vi "Main GNSS-w-Ntrip.vi"() -> ()   [LabVIEW 2019]
uses:
  C:/Users/WEGO/Documents/GitHub/Ycar/LabVIEW/Gmap/dll/GMap.NET.WindowsForms.dll
  Gmap/dll/GMap.NET.WindowsForms.dll
  Ctrl/ublox-ui_main.ctl
  Ctrl/gnss_config-2.ctl
  Ctrl/cmd_ini-add-read.ctl
  Ctrl/cmd_ini-RW.ctl
  Ctrl/cmd_common.ctl
  Ctrl/GNSS-Ntrip config.ctl
  Gmap/gmap_fgv-cmd.ctl
  Ctrl/cmd_RW.ctl
panel:
  out "GNSS time":string
  out "Ntrip conn":bool
  out "NMEA val":bool
  in  "main tap":T1(tab)
  in  "Serial Send Start/Stop":bool
  in  "GNSS Start/Stop":bool
  out "TM\nptn":u32(slide) scale=0.0..200.0
  in  "Local Time offset":u32=9
  in  "GMapControl":refnum<k24>(container)
  out "Sea Level":dbl
  out "N of Satellites":i32
  out "TM graph":T2(graph)=[{"TM array"=[{"Y(E)"=195478.83340938148, "X(N)"=532749.6315443226}, {"Y(E)"=195478.83340938148, "X(N)"=532749.6315443226}, {"Y(E)"=195478.83340938148, "X(N)"=532749.6315443226}, {"Y(E)"=195478.83340938148, "X(N)"=532749.6315443226}, {"Y(E)"=195478.83340938148, "X(N)"=532749.6315443226}, {"Y(E)"=195478.83340938148, "X(N)"=532749.6315443226}, {"Y(E)"=195478.83340938148, "X(N)"=532749.6315443226}, {"Y(E)"=195478.83340938148, "X(N)"=532749.6315443226}, {"Y(E)"=195478.83340938148, "X(N)"=532749.6315443226}, {"Y(E)"=195478.83340938148, "X(N)"=532749.6315443226}, {"Y(E)"=195478.80387262133, "X(N)"=532749.5945652778}, {"Y(E)"=195478.80387262133, "X(N)"=532749.5945652778}, {"Y(E)"=195478.80387262133, "X(N)"=532749.5945652778}, {"Y(E)"=195478.80387262133, "X(N)"=532749.5945652778}, {"Y(E)"=195478.80387262133, "X(N)"=532749.5945652778}, {"Y(E)"=195478.80387262133, "X(N)"=532749.5945652778}, {"Y(E)"=195478.80387262133, "X(N)"=532749.5945652778}, {"Y(E)"=195478.80387262133, "X(N)"=532749.5945652778}, {"Y(E)"=195478.80387262133, "X(N)"=532749.5945652778}, {"Y(E)"=195478.80387262133, "X(N)"=532749.5945652778}, {"Y(E)"=195478.80387262133, "X(N)"=532749.5945652778}, {"Y(E)"=195478.80387262133, "X(N)"=532749.5945652778}, {"Y(E)"=195478.80387262133, "X(N)"=532749.5945652778}, {"Y(E)"=195478.86283602339, "X(N)"=532749.4650507653}, {"Y(E)"=195478.86283602339, "X(N)"=532749.4650507653}, {"Y(E)"=195478.86283602339, "X(N)"=532749.4650507653}, {"Y(E)"=195478.86283602339, "X(N)"=532749.4650507653}, {"Y(E)"=195478.86283602339, "X(N)"=532749.4650507653}, {"Y(E)"=195478.86283602339, "X(N)"=532749.4650507653}, {"Y(E)"=195478.86283602339, "X(N)"=532749.4650507653}, {"Y(E)"=195478.86283602339, "X(N)"=532749.4650507653}, {"Y(E)"=195478.86283602339, "X(N)"=532749.4650507653}, {"Y(E)"=195478.86283602339, "X(N)"=532749.4650507653}, {"Y(E)"=195478.86283602339, "X(N)"=532749.4650507653}, {"Y(E)"=195478.86283602339, "X(N)"=532749.4650507653}, {"Y(E)"=195478.86283602339, "X(N)"=532749.4650507653}, {"Y(E)"=195478.8185809412, "X(N)"=532749.5020697443}, {"Y(E)"=195478.8185809412, "X(N)"=532749.5020697443}, {"Y(E)"=195478.8185809412, "X(N)"=532749.5020697443}, {"Y(E)"=195478.8185809412, "X(N)"=532749.5020697443}, {"Y(E)"=195478.8185809412, "X(N)"=532749.5020697443}, {"Y(E)"=195478.8185809412, "X(N)"=532749.5020697443}, {"Y(E)"=195478.8185809412, "X(N)"=532749.5020697443}, {"Y(E)"=195478.8185809412, "X(N)"=532749.5020697443}, {"Y(E)"=195478.8185809412, "X(N)"=532749.5020697443}, {"Y(E)"=195478.8185809412, "X(N)"=532749.5020697443}, {"Y(E)"=195478.8185809412, "X(N)"=532749.5020697443}, {"Y(E)"=195478.8185809412, "X(N)"=532749.5020697443}, {"Y(E)"=195478.8185809412, "X(N)"=532749.5020697443}, {"Y(E)"=195478.8333493192, "X(N)"=532749.5205592669}, {"Y(E)"=195478.8333493192, "X(N)"=532749.5205592669}, {"Y(E)"=195478.8333493192, "X(N)"=532749.5205592669}, {"Y(E)"=195478.8333493192, "X(N)"=532749.5205592669}, {"Y(E)"=195478.8333493192, "X(N)"=532749.5205592669}, {"Y(E)"=195478.8333493192, "X(N)"=532749.5205592669}, {"Y(E)"=195478.8333493192, "X(N)"=532749.5205592669}, {"Y(E)"=195478.8333493192, "X(N)"=532749.5205592669}, {"Y(E)"=195478.8333493192, "X(N)"=532749.5205592669}, {"Y(E)"=195478.8333493192, "X(N)"=532749.5205592669}, {"Y(E)"=195478.8333493192, "X(N)"=532749.5205592669}, {"Y(E)"=195478.8333493192, "X(N)"=532749.5205592669}, {"Y(E)"=195478.81854089958, "X(N)"=532749.4280797082}, {"Y(E)"=195478.81854089958, "X(N)"=532749.4280797082}, {"Y(E)"=195478.81854089958, "X(N)"=532749.4280797082}, {"Y(E)"=195478.81854089958, "X(N)"=532749.4280797082}, {"Y(E)"=195478.81854089958, "X(N)"=532749.4280797082}, {"Y(E)"=195478.81854089958, "X(N)"=532749.4280797082}, {"Y(E)"=195478.81854089958, "X(N)"=532749.4280797082}, {"Y(E)"=195478.81854089958, "X(N)"=532749.4280797082}, {"Y(E)"=195478.81854089958, "X(N)"=532749.4280797082}, {"Y(E)"=195478.81854089958, "X(N)"=532749.4280797082}, {"Y(E)"=195478.81854089958, "X(N)"=532749.4280797082}, {"Y(E)"=195478.81854089958, "X(N)"=532749.4280797082}, {"Y(E)"=195478.81854089958, "X(N)"=532749.4280797082}, {"Y(E)"=195478.8332592258, "X(N)"=532749.3540816847}, {"Y(E)"=195478.8332592258, "X(N)"=532749.3540816847}, {"Y(E)"=195478.8332592258, "X(N)"=532749.3540816847}, {"Y(E)"=195478.8332592258, "X(N)"=532749.3540816847}, {"Y(E)"=195478.8332592258, "X(N)"=532749.3540816847}, {"Y(E)"=195478.8332592258, "X(N)"=532749.3540816847}, {"Y(E)"=195478.8332592258, "X(N)"=532749.3540816847}, {"Y(E)"=195478.8332592258, "X(N)"=532749.3540816847}, {"Y(E)"=195478.8332592258, "X(N)"=532749.3540816847}, {"Y(E)"=195478.8332592258, "X(N)"=532749.3540816847}, {"Y(E)"=195478.8332592258, "X(N)"=532749.3540816847}, {"Y(E)"=195478.8332592258, "X(N)"=532749.3540816847}, {"Y(E)"=195478.8332592258, "X(N)"=532749.3540816847}, {"Y(E)"=195478.61200383154, "X(N)"=532749.5761715989}, {"Y(E)"=195478.61200383154, "X(N)"=532749.5761715989}, {"Y(E)"=195478.61200383154, "X(N)"=532749.5761715989}, {"Y(E)"=195478.61200383154, "X(N)"=532749.5761715989}, {"Y(E)"=195478.61200383154, "X(N)"=532749.5761715989}, {"Y(E)"=195478.61200383154, "X(N)"=532749.5761715989}, {"Y(E)"=195478.61200383154, "X(N)"=532749.5761715989}, {"Y(E)"=195478.61200383154, "X(N)"=532749.5761715989}, {"Y(E)"=195478.61200383154, "X(N)"=532749.5761715989}, {"Y(E)"=195478.61200383154, "X(N)"=532749.5761715989}, {"Y(E)"=195478.61200383154, "X(N)"=532749.5761715989}, {"Y(E)"=195478.61200383154, "X(N)"=532749.5761715989}, {"Y(E)"=195478.61200383154, "X(N)"=532749.5761715989}, {"Y(E)"=195478.61197379892, "X(N)"=532749.5206790727}, {"Y(E)"=195478.61197379892, "X(N)"=532749.5206790727}, {"Y(E)"=195478.61197379892, "X(N)"=532749.5206790727}, {"Y(E)"=195478.61197379892, "X(N)"=532749.5206790727}, {"Y(E)"=195478.61197379892, "X(N)"=532749.5206790727}, {"Y(E)"=195478.61197379892, "X(N)"=532749.5206790727}, {"Y(E)"=195478.61197379892, "X(N)"=532749.5206790727}, {"Y(E)"=195478.61197379892, "X(N)"=532749.5206790727}, {"Y(E)"=195478.61197379892, "X(N)"=532749.5206790727}, {"Y(E)"=195478.61197379892, "X(N)"=532749.5206790727}, {"Y(E)"=195478.61197379892, "X(N)"=532749.5206790727}, {"Y(E)"=195478.61197379892, "X(N)"=532749.5206790727}, {"Y(E)"=195478.61197379892, "X(N)"=532749.5206790727}, {"Y(E)"=195478.64144048005, "X(N)"=532749.4281755526}, {"Y(E)"=195478.64144048005, "X(N)"=532749.4281755526}, {"Y(E)"=195478.64144048005, "X(N)"=532749.4281755526}, {"Y(E)"=195478.64144048005, "X(N)"=532749.4281755526}, {"Y(E)"=195478.64144048005, "X(N)"=532749.4281755526}, {"Y(E)"=195478.64144048005, "X(N)"=532749.4281755526}, {"Y(E)"=195478.64144048005, "X(N)"=532749.4281755526}, {"Y(E)"=195478.64144048005, "X(N)"=532749.4281755526}, {"Y(E)"=195478.64144048005, "X(N)"=532749.4281755526}, {"Y(E)"=195478.64144048005, "X(N)"=532749.4281755526}, {"Y(E)"=195478.64144048005, "X(N)"=532749.4281755526}, {"Y(E)"=195478.64144048005, "X(N)"=532749.4281755526}, {"Y(E)"=195478.64144048005, "X(N)"=532749.4281755526}, {"Y(E)"=195478.56754852948, "X(N)"=532749.2432403986}, {"Y(E)"=195478.56754852948, "X(N)"=532749.2432403986}, {"Y(E)"=195478.56754852948, "X(N)"=532749.2432403986}, {"Y(E)"=195478.56754852948, "X(N)"=532749.2432403986}, {"Y(E)"=195478.56754852948, "X(N)"=532749.2432403986}, {"Y(E)"=195478.56754852948, "X(N)"=532749.2432403986}, {"Y(E)"=195478.56754852948, "X(N)"=532749.2432403986}, {"Y(E)"=195478.56754852948, "X(N)"=532749.2432403986}, {"Y(E)"=195478.56754852948, "X(N)"=532749.2432403986}, {"Y(E)"=195478.56754852948, "X(N)"=532749.2432403986}, {"Y(E)"=195478.56754852948, "X(N)"=532749.2432403986}, {"Y(E)"=195478.56754852948, "X(N)"=532749.2432403986}, {"Y(E)"=195478.56754852948, "X(N)"=532749.2432403986}, {"Y(E)"=195478.5822568451, "X(N)"=532749.1507448669}, {"Y(E)"=195478.5822568451, "X(N)"=532749.1507448669}, {"Y(E)"=195478.5822568451, "X(N)"=532749.1507448669}, {"Y(E)"=195478.5822568451, "X(N)"=532749.1507448669}, {"Y(E)"=195478.5822568451, "X(N)"=532749.1507448669}, {"Y(E)"=195478.5822568451, "X(N)"=532749.1507448669}, {"Y(E)"=195478.5822568451, "X(N)"=532749.1507448669}, {"Y(E)"=195478.5822568451, "X(N)"=532749.1507448669}, {"Y(E)"=195478.5822568451, "X(N)"=532749.1507448669}, {"Y(E)"=195478.5822568451, "X(N)"=532749.1507448669}, {"Y(E)"=195478.5822568451, "X(N)"=532749.1507448669}, {"Y(E)"=195478.5822568451, "X(N)"=532749.1507448669}, {"Y(E)"=195478.5822568451, "X(N)"=532749.1507448669}, {"Y(E)"=195478.3755095352, "X(N)"=532748.9103890732}, {"Y(E)"=195478.3755095352, "X(N)"=532748.9103890732}, {"Y(E)"=195478.3755095352, "X(N)"=532748.9103890732}, {"Y(E)"=195478.3755095352, "X(N)"=532748.9103890732}, {"Y(E)"=195478.3755095352, "X(N)"=532748.9103890732}, {"Y(E)"=195478.3755095352, "X(N)"=532748.9103890732}, {"Y(E)"=195478.3755095352, "X(N)"=532748.9103890732}, {"Y(E)"=195478.3755095352, "X(N)"=532748.9103890732}, {"Y(E)"=195478.3755095352, "X(N)"=532748.9103890732}, {"Y(E)"=195478.3755095352, "X(N)"=532748.9103890732}, {"Y(E)"=195478.3755095352, "X(N)"=532748.9103890732}, {"Y(E)"=195478.3755095352, "X(N)"=532748.9103890732}, {"Y(E)"=195478.3755095352, "X(N)"=532748.9103890732}, {"Y(E)"=195478.37543945547, "X(N)"=532748.78090651}, {"Y(E)"=195478.37543945547, "X(N)"=532748.78090651}, {"Y(E)"=195478.37543945547, "X(N)"=532748.78090651}, {"Y(E)"=195478.37543945547, "X(N)"=532748.78090651}, {"Y(E)"=195478.37543945547, "X(N)"=532748.78090651}, {"Y(E)"=195478.37543945547, "X(N)"=532748.78090651}, {"Y(E)"=195478.37543945547, "X(N)"=532748.78090651}, {"Y(E)"=195478.37543945547, "X(N)"=532748.78090651}, {"Y(E)"=195478.37543945547, "X(N)"=532748.78090651}, {"Y(E)"=195478.37543945547, "X(N)"=532748.78090651}, {"Y(E)"=195478.37543945547, "X(N)"=532748.78090651}, {"Y(E)"=195478.37543945547, "X(N)"=532748.78090651}, {"Y(E)"=195478.5082848043, "X(N)"=532748.8178296402}, {"Y(E)"=195478.5082848043, "X(N)"=532748.8178296402}, {"Y(E)"=195478.5082848043, "X(N)"=532748.8178296402}, {"Y(E)"=195478.5082848043, "X(N)"=532748.8178296402}, {"Y(E)"=195478.5082848043, "X(N)"=532748.8178296402}, {"Y(E)"=195478.5082848043, "X(N)"=532748.8178296402}, {"Y(E)"=195478.5082848043, "X(N)"=532748.8178296402}, {"Y(E)"=195478.5082848043, "X(N)"=532748.8178296402}, {"Y(E)"=195478.5082848043, "X(N)"=532748.8178296402}, {"Y(E)"=195478.5082848043, "X(N)"=532748.8178296402}, {"Y(E)"=195478.5082848043, "X(N)"=532748.8178296402}, {"Y(E)"=195478.5082848043, "X(N)"=532748.8178296402}, {"Y(E)"=195478.5082848043, "X(N)"=532748.8178296402}, {"Y(E)"=195478.7001636224, "X(N)"=532748.8547208244}, {"Y(E)"=195478.7001636224, "X(N)"=532748.8547208244}, {"Y(E)"=195478.7001636224, "X(N)"=532748.8547208244}, {"Y(E)"=195478.7001636224, "X(N)"=532748.8547208244}, {"Y(E)"=195478.7001636224, "X(N)"=532748.8547208244}, {"Y(E)"=195478.7001636224, "X(N)"=532748.8547208244}, {"Y(E)"=195478.7001636224, "X(N)"=532748.8547208244}, {"Y(E)"=195478.7001636224, "X(N)"=532748.8547208244}, {"Y(E)"=195478.7001636224, "X(N)"=532748.8547208244}, {"Y(E)"=195478.7001636224, "X(N)"=532748.8547208244}]}, {"TM array"=[{"Y(E)"=195478.60442441847, "X(N)"=532749.6892681528}, {"Y(E)"=195478.63475492285, "X(N)"=532749.6883149784}, {"Y(E)"=195478.6649657266, "X(N)"=532749.6854592166}, {"Y(E)"=195478.69493760145, "X(N)"=532749.680712138}, {"Y(E)"=195478.72455226214, "X(N)"=532749.6740924771}, {"Y(E)"=195478.7536928331, "X(N)"=532749.6656263586}, {"Y(E)"=195478.7822443098, "X(N)"=532749.6553471944}, {"Y(E)"=195478.81009401265, "X(N)"=532749.6432955518}, {"Y(E)"=195478.83713203156, "X(N)"=532749.6295189931}, {"Y(E)"=195478.86325165984, "X(N)"=532749.6140718879}, {"Y(E)"=195478.88834981524, "X(N)"=532749.5970151991}, {"Y(E)"=195478.91232744683, "X(N)"=532749.5784162417}, {"Y(E)"=195478.93508992583, "X(N)"=532749.5583484169}, {"Y(E)"=195478.95654741913, "X(N)"=532749.5368909236}, {"Y(E)"=195478.97661524382, "X(N)"=532749.5141284446}, {"Y(E)"=195478.99521420136, "X(N)"=532749.490150813}, {"Y(E)"=195479.01227089018, "X(N)"=532749.4650526576}, {"Y(E)"=195479.02771799528, "X(N)"=532749.4389330294}, {"Y(E)"=195479.04149455403, "X(N)"=532749.4118950105}, {"Y(E)"=195479.0535461966, "X(N)"=532749.3840453076}, {"Y(E)"=195479.06382536073, "X(N)"=532749.3554938309}, {"Y(E)"=195479.0722914792, "X(N)"=532749.32635326}, {"Y(E)"=195479.07891114015, "X(N)"=532749.2967385993}, {"Y(E)"=195479.0836582188, "X(N)"=532749.2667667244}, {"Y(E)"=195479.08651398055, "X(N)"=532749.2365559207}, {"Y(E)"=195479.08746715504, "X(N)"=532749.2062254163}, {"Y(E)"=195479.08651398055, "X(N)"=532749.1758949119}, {"Y(E)"=195479.0836582188, "X(N)"=532749.1456841081}, {"Y(E)"=195479.07891114015, "X(N)"=532749.1157122332}, {"Y(E)"=195479.0722914792, "X(N)"=532749.0860975726}, {"Y(E)"=195479.06382536073, "X(N)"=532749.0569570017}, {"Y(E)"=195479.0535461966, "X(N)"=532749.0284055249}, {"Y(E)"=195479.04149455403, "X(N)"=532749.000555822}, {"Y(E)"=195479.02771799528, "X(N)"=532748.9735178031}, {"Y(E)"=195479.01227089018, "X(N)"=532748.9473981749}, {"Y(E)"=195478.99521420136, "X(N)"=532748.9223000195}, {"Y(E)"=195478.97661524382, "X(N)"=532748.898322388}, {"Y(E)"=195478.95654741913, "X(N)"=532748.8755599089}, {"Y(E)"=195478.93508992583, "X(N)"=532748.8541024156}, {"Y(E)"=195478.91232744683, "X(N)"=532748.8340345909}, {"Y(E)"=195478.88834981524, "X(N)"=532748.8154356334}, {"Y(E)"=195478.86325165984, "X(N)"=532748.7983789446}, {"Y(E)"=195478.83713203156, "X(N)"=532748.7829318395}, {"Y(E)"=195478.81009401265, "X(N)"=532748.7691552808}, {"Y(E)"=195478.7822443098, "X(N)"=532748.7571036381}, {"Y(E)"=195478.7536928331, "X(N)"=532748.746824474}, {"Y(E)"=195478.72455226214, "X(N)"=532748.7383583555}, {"Y(E)"=195478.69493760145, "X(N)"=532748.7317386946}, {"Y(E)"=195478.6649657266, "X(N)"=532748.726991616}, {"Y(E)"=195478.63475492285, "X(N)"=532748.7241358542}, {"Y(E)"=195478.60442441847, "X(N)"=532748.7231826797}, {"Y(E)"=195478.5740939141, "X(N)"=532748.7241358542}, {"Y(E)"=195478.54388311034, "X(N)"=532748.726991616}, {"Y(E)"=195478.5139112355, "X(N)"=532748.7317386946}, {"Y(E)"=195478.4842965748, "X(N)"=532748.7383583555}, {"Y(E)"=195478.45515600385, "X(N)"=532748.746824474}, {"Y(E)"=195478.42660452714, "X(N)"=532748.7571036381}, {"Y(E)"=195478.3987548243, "X(N)"=532748.7691552808}, {"Y(E)"=195478.37171680538, "X(N)"=532748.7829318395}, {"Y(E)"=195478.3455971771, "X(N)"=532748.7983789446}, {"Y(E)"=195478.3204990217, "X(N)"=532748.8154356334}, {"Y(E)"=195478.29652139012, "X(N)"=532748.8340345909}, {"Y(E)"=195478.27375891112, "X(N)"=532748.8541024156}, {"Y(E)"=195478.25230141782, "X(N)"=532748.8755599089}, {"Y(E)"=195478.23223359312, "X(N)"=532748.898322388}, {"Y(E)"=195478.21363463558, "X(N)"=532748.9223000195}, {"Y(E)"=195478.19657794677, "X(N)"=532748.9473981749}, {"Y(E)"=195478.18113084167, "X(N)"=532748.9735178031}, {"Y(E)"=195478.16735428292, "X(N)"=532749.000555822}, {"Y(E)"=195478.15530264034, "X(N)"=532749.0284055249}, {"Y(E)"=195478.14502347622, "X(N)"=532749.0569570017}, {"Y(E)"=195478.13655735774, "X(N)"=532749.0860975726}, {"Y(E)"=195478.1299376968, "X(N)"=532749.1157122332}, {"Y(E)"=195478.12519061816, "X(N)"=532749.1456841081}, {"Y(E)"=195478.1223348564, "X(N)"=532749.1758949119}, {"Y(E)"=195478.1213816819, "X(N)"=532749.2062254163}, {"Y(E)"=195478.1223348564, "X(N)"=532749.2365559207}, {"Y(E)"=195478.12519061816, "X(N)"=532749.2667667244}, {"Y(E)"=195478.1299376968, "X(N)"=532749.2967385993}, {"Y(E)"=195478.13655735774, "X(N)"=532749.32635326}, {"Y(E)"=195478.14502347622, "X(N)"=532749.3554938309}, {"Y(E)"=195478.15530264034, "X(N)"=532749.3840453076}, {"Y(E)"=195478.16735428292, "X(N)"=532749.4118950105}, {"Y(E)"=195478.18113084167, "X(N)"=532749.4389330294}, {"Y(E)"=195478.19657794677, "X(N)"=532749.4650526576}, {"Y(E)"=195478.21363463558, "X(N)"=532749.490150813}, {"Y(E)"=195478.23223359312, "X(N)"=532749.5141284446}, {"Y(E)"=195478.25230141782, "X(N)"=532749.5368909236}, {"Y(E)"=195478.27375891112, "X(N)"=532749.5583484169}, {"Y(E)"=195478.29652139012, "X(N)"=532749.5784162417}, {"Y(E)"=195478.3204990217, "X(N)"=532749.5970151991}, {"Y(E)"=195478.3455971771, "X(N)"=532749.6140718879}, {"Y(E)"=195478.37171680538, "X(N)"=532749.6295189931}, {"Y(E)"=195478.3987548243, "X(N)"=532749.6432955518}, {"Y(E)"=195478.42660452714, "X(N)"=532749.6553471944}, {"Y(E)"=195478.45515600385, "X(N)"=532749.6656263586}, {"Y(E)"=195478.4842965748, "X(N)"=532749.6740924771}, {"Y(E)"=195478.5139112355, "X(N)"=532749.680712138}, {"Y(E)"=195478.54388311034, "X(N)"=532749.6854592166}, {"Y(E)"=195478.5740939141, "X(N)"=532749.6883149784}, {"Y(E)"=195478.60442441847, "X(N)"=532749.6892681528}]}, {"TM array"=[{"Y(E)"=195478.60442441847, "X(N)"=532750.2062254163}, {"Y(E)"=195478.667214938, "X(N)"=532750.2042521447}, {"Y(E)"=195478.72975765204, "X(N)"=532750.1983401176}, {"Y(E)"=195478.79180573305, "X(N)"=532750.188512667}, {"Y(E)"=195478.85311430565, "X(N)"=532750.1748085774}, {"Y(E)"=195478.91344141285, "X(N)"=532750.1572819325}, {"Y(E)"=195478.97254897116, "X(N)"=532750.1360019022}, {"Y(E)"=195479.03020371005, "X(N)"=532750.1110524688}, {"Y(E)"=195479.08617809258, "X(N)"=532750.0825320963}, {"Y(E)"=195479.14025121345, "X(N)"=532750.0505533417}, {"Y(E)"=195479.19220967076, "X(N)"=532750.0152424106}, {"Y(E)"=195479.24184840822, "X(N)"=532749.9767386591}, {"Y(E)"=195479.2889715244, "X(N)"=532749.9351940437}, {"Y(E)"=195479.3333930459, "X(N)"=532749.8907725222}, {"Y(E)"=195479.37493766125, "X(N)"=532749.843649406}, {"Y(E)"=195479.41344141285, "X(N)"=532749.7940106685}, {"Y(E)"=195479.44875234397, "X(N)"=532749.7420522113}, {"Y(E)"=195479.4807310985, "X(N)"=532749.6879790904}, {"Y(E)"=195479.50925147094, "X(N)"=532749.6320047078}, {"Y(E)"=195479.53420090437, "X(N)"=532749.5743499689}, {"Y(E)"=195479.55548093477, "X(N)"=532749.5152424106}, {"Y(E)"=195479.5730075796, "X(N)"=532749.4549153034}, {"Y(E)"=195479.5867116692, "X(N)"=532749.3936067309}, {"Y(E)"=195479.59653911978, "X(N)"=532749.3315586499}, {"Y(E)"=195479.6024511469, "X(N)"=532749.2690159358}, {"Y(E)"=195479.60442441847, "X(N)"=532749.2062254163}, {"Y(E)"=195479.6024511469, "X(N)"=532749.1434348967}, {"Y(E)"=195479.59653911978, "X(N)"=532749.0808921827}, {"Y(E)"=195479.5867116692, "X(N)"=532749.0188441017}, {"Y(E)"=195479.5730075796, "X(N)"=532748.9575355292}, {"Y(E)"=195479.55548093477, "X(N)"=532748.897208422}, {"Y(E)"=195479.53420090437, "X(N)"=532748.8381008636}, {"Y(E)"=195479.50925147094, "X(N)"=532748.7804461247}, {"Y(E)"=195479.4807310985, "X(N)"=532748.7244717422}, {"Y(E)"=195479.44875234397, "X(N)"=532748.6703986212}, {"Y(E)"=195479.41344141285, "X(N)"=532748.618440164}, {"Y(E)"=195479.37493766125, "X(N)"=532748.5688014266}, {"Y(E)"=195479.3333930459, "X(N)"=532748.5216783104}, {"Y(E)"=195479.2889715244, "X(N)"=532748.4772567889}, {"Y(E)"=195479.24184840822, "X(N)"=532748.4357121735}, {"Y(E)"=195479.19220967076, "X(N)"=532748.397208422}, {"Y(E)"=195479.14025121345, "X(N)"=532748.3618974908}, {"Y(E)"=195479.08617809258, "X(N)"=532748.3299187362}, {"Y(E)"=195479.03020371005, "X(N)"=532748.3013983638}, {"Y(E)"=195478.97254897116, "X(N)"=532748.2764489304}, {"Y(E)"=195478.91344141285, "X(N)"=532748.2551689}, {"Y(E)"=195478.85311430565, "X(N)"=532748.2376422551}, {"Y(E)"=195478.79180573305, "X(N)"=532748.2239381656}, {"Y(E)"=195478.72975765204, "X(N)"=532748.214110715}, {"Y(E)"=195478.667214938, "X(N)"=532748.2081986879}, {"Y(E)"=195478.60442441847, "X(N)"=532748.2062254163}, {"Y(E)"=195478.54163389895, "X(N)"=532748.2081986879}, {"Y(E)"=195478.4790911849, "X(N)"=532748.214110715}, {"Y(E)"=195478.4170431039, "X(N)"=532748.2239381656}, {"Y(E)"=195478.3557345313, "X(N)"=532748.2376422551}, {"Y(E)"=195478.2954074241, "X(N)"=532748.2551689}, {"Y(E)"=195478.2362998658, "X(N)"=532748.2764489304}, {"Y(E)"=195478.1786451269, "X(N)"=532748.3013983638}, {"Y(E)"=195478.12267074437, "X(N)"=532748.3299187362}, {"Y(E)"=195478.0685976235, "X(N)"=532748.3618974908}, {"Y(E)"=195478.0166391662, "X(N)"=532748.397208422}, {"Y(E)"=195477.96700042873, "X(N)"=532748.4357121735}, {"Y(E)"=195477.91987731255, "X(N)"=532748.4772567889}, {"Y(E)"=195477.87545579104, "X(N)"=532748.5216783104}, {"Y(E)"=195477.8339111757, "X(N)"=532748.5688014266}, {"Y(E)"=195477.7954074241, "X(N)"=532748.618440164}, {"Y(E)"=195477.76009649297, "X(N)"=532748.6703986212}, {"Y(E)"=195477.72811773844, "X(N)"=532748.7244717422}, {"Y(E)"=195477.699597366, "X(N)"=532748.7804461247}, {"Y(E)"=195477.67464793258, "X(N)"=532748.8381008636}, {"Y(E)"=195477.65336790218, "X(N)"=532748.897208422}, {"Y(E)"=195477.63584125735, "X(N)"=532748.9575355292}, {"Y(E)"=195477.62213716775, "X(N)"=532749.0188441017}, {"Y(E)"=195477.61230971717, "X(N)"=532749.0808921827}, {"Y(E)"=195477.60639769005, "X(N)"=532749.1434348967}, {"Y(E)"=195477.60442441847, "X(N)"=532749.2062254163}, {"Y(E)"=195477.60639769005, "X(N)"=532749.2690159358}, {"Y(E)"=195477.61230971717, "X(N)"=532749.3315586499}, {"Y(E)"=195477.62213716775, "X(N)"=532749.3936067309}, {"Y(E)"=195477.63584125735, "X(N)"=532749.4549153034}, {"Y(E)"=195477.65336790218, "X(N)"=532749.5152424106}, {"Y(E)"=195477.67464793258, "X(N)"=532749.5743499689}, {"Y(E)"=195477.699597366, "X(N)"=532749.6320047078}, {"Y(E)"=195477.72811773844, "X(N)"=532749.6879790904}, {"Y(E)"=195477.76009649297, "X(N)"=532749.7420522113}, {"Y(E)"=195477.7954074241, "X(N)"=532749.7940106685}, {"Y(E)"=195477.8339111757, "X(N)"=532749.843649406}, {"Y(E)"=195477.87545579104, "X(N)"=532749.8907725222}, {"Y(E)"=195477.91987731255, "X(N)"=532749.9351940437}, {"Y(E)"=195477.96700042873, "X(N)"=532749.9767386591}, {"Y(E)"=195478.0166391662, "X(N)"=532750.0152424106}, {"Y(E)"=195478.0685976235, "X(N)"=532750.0505533417}, {"Y(E)"=195478.12267074437, "X(N)"=532750.0825320963}, {"Y(E)"=195478.1786451269, "X(N)"=532750.1110524688}, {"Y(E)"=195478.2362998658, "X(N)"=532750.1360019022}, {"Y(E)"=195478.2954074241, "X(N)"=532750.1572819325}, {"Y(E)"=195478.3557345313, "X(N)"=532750.1748085774}, {"Y(E)"=195478.4170431039, "X(N)"=532750.188512667}, {"Y(E)"=195478.4790911849, "X(N)"=532750.1983401176}, {"Y(E)"=195478.54163389895, "X(N)"=532750.2042521447}, {"Y(E)"=195478.60442441847, "X(N)"=532750.2062254163}]}, {"TM array"=[{"Y(E)"=195478.60442441847, "X(N)"=532751.2062254163}, {"Y(E)"=195478.73000545753, "X(N)"=532751.2022788732}, {"Y(E)"=195478.8550908856, "X(N)"=532751.1904548189}, {"Y(E)"=195478.97918704763, "X(N)"=532751.1707999178}, {"Y(E)"=195479.10180419282, "X(N)"=532751.1433917385}, {"Y(E)"=195479.22245840722, "X(N)"=532751.1083384489}, {"Y(E)"=195479.34067352384, "X(N)"=532751.0657783881}, {"Y(E)"=195479.4559830016, "X(N)"=532751.0158795213}, {"Y(E)"=195479.56793176668, "X(N)"=532750.9588387763}, {"Y(E)"=195479.67607800843, "X(N)"=532750.8948812673}, {"Y(E)"=195479.77999492307, "X(N)"=532750.824259405}, {"Y(E)"=195479.879272398, "X(N)"=532750.7472519018}, {"Y(E)"=195479.97351863034, "X(N)"=532750.6641626711}, {"Y(E)"=195480.0623616733, "X(N)"=532750.5753196281}, {"Y(E)"=195480.14545090403, "X(N)"=532750.4810733958}, {"Y(E)"=195480.22245840722, "X(N)"=532750.3817959209}, {"Y(E)"=195480.29308026948, "X(N)"=532750.2778790062}, {"Y(E)"=195480.35703777857, "X(N)"=532750.1697327645}, {"Y(E)"=195480.4140785234, "X(N)"=532750.0577839994}, {"Y(E)"=195480.46397739026, "X(N)"=532749.9424745217}, {"Y(E)"=195480.50653745106, "X(N)"=532749.824259405}, {"Y(E)"=195480.54159074073, "X(N)"=532749.7036051906}, {"Y(E)"=195480.56899891995, "X(N)"=532749.5809880454}, {"Y(E)"=195480.5886538211, "X(N)"=532749.4568918834}, {"Y(E)"=195480.60047787533, "X(N)"=532749.3318064554}, {"Y(E)"=195480.60442441847, "X(N)"=532749.2062254163}, {"Y(E)"=195480.60047787533, "X(N)"=532749.0806443772}, {"Y(E)"=195480.5886538211, "X(N)"=532748.9555589492}, {"Y(E)"=195480.56899891995, "X(N)"=532748.8314627871}, {"Y(E)"=195480.54159074073, "X(N)"=532748.7088456419}, {"Y(E)"=195480.50653745106, "X(N)"=532748.5881914275}, {"Y(E)"=195480.46397739026, "X(N)"=532748.4699763109}, {"Y(E)"=195480.4140785234, "X(N)"=532748.3546668332}, {"Y(E)"=195480.35703777857, "X(N)"=532748.2427180681}, {"Y(E)"=195480.29308026948, "X(N)"=532748.1345718263}, {"Y(E)"=195480.22245840722, "X(N)"=532748.0306549117}, {"Y(E)"=195480.14545090403, "X(N)"=532747.9313774367}, {"Y(E)"=195480.0623616733, "X(N)"=532747.8371312044}, {"Y(E)"=195479.97351863034, "X(N)"=532747.7482881615}, {"Y(E)"=195479.879272398, "X(N)"=532747.6651989308}, {"Y(E)"=195479.77999492307, "X(N)"=532747.5881914275}, {"Y(E)"=195479.67607800843, "X(N)"=532747.5175695652}, {"Y(E)"=195479.56793176668, "X(N)"=532747.4536120562}, {"Y(E)"=195479.4559830016, "X(N)"=532747.3965713113}, {"Y(E)"=195479.34067352384, "X(N)"=532747.3466724445}, {"Y(E)"=195479.22245840722, "X(N)"=532747.3041123836}, {"Y(E)"=195479.10180419282, "X(N)"=532747.269059094}, {"Y(E)"=195478.97918704763, "X(N)"=532747.2416509148}, {"Y(E)"=195478.8550908856, "X(N)"=532747.2219960137}, {"Y(E)"=195478.73000545753, "X(N)"=532747.2101719594}, {"Y(E)"=195478.60442441847, "X(N)"=532747.2062254163}, {"Y(E)"=195478.47884337942, "X(N)"=532747.2101719594}, {"Y(E)"=195478.35375795135, "X(N)"=532747.2219960137}, {"Y(E)"=195478.22966178932, "X(N)"=532747.2416509148}, {"Y(E)"=195478.10704464413, "X(N)"=532747.269059094}, {"Y(E)"=195477.98639042972, "X(N)"=532747.3041123836}, {"Y(E)"=195477.8681753131, "X(N)"=532747.3466724445}, {"Y(E)"=195477.75286583535, "X(N)"=532747.3965713113}, {"Y(E)"=195477.64091707027, "X(N)"=532747.4536120562}, {"Y(E)"=195477.53277082852, "X(N)"=532747.5175695652}, {"Y(E)"=195477.42885391388, "X(N)"=532747.5881914275}, {"Y(E)"=195477.32957643896, "X(N)"=532747.6651989308}, {"Y(E)"=195477.2353302066, "X(N)"=532747.7482881615}, {"Y(E)"=195477.14648716364, "X(N)"=532747.8371312044}, {"Y(E)"=195477.0633979329, "X(N)"=532747.9313774367}, {"Y(E)"=195476.98639042972, "X(N)"=532748.0306549117}, {"Y(E)"=195476.91576856747, "X(N)"=532748.1345718263}, {"Y(E)"=195476.85181105838, "X(N)"=532748.2427180681}, {"Y(E)"=195476.79477031354, "X(N)"=532748.3546668332}, {"Y(E)"=195476.7448714467, "X(N)"=532748.4699763109}, {"Y(E)"=195476.7023113859, "X(N)"=532748.5881914275}, {"Y(E)"=195476.66725809622, "X(N)"=532748.7088456419}, {"Y(E)"=195476.639849917, "X(N)"=532748.8314627871}, {"Y(E)"=195476.62019501586, "X(N)"=532748.9555589492}, {"Y(E)"=195476.60837096162, "X(N)"=532749.0806443772}, {"Y(E)"=195476.60442441847, "X(N)"=532749.2062254163}, {"Y(E)"=195476.60837096162, "X(N)"=532749.3318064554}, {"Y(E)"=195476.62019501586, "X(N)"=532749.4568918834}, {"Y(E)"=195476.639849917, "X(N)"=532749.5809880454}, {"Y(E)"=195476.66725809622, "X(N)"=532749.7036051906}, {"Y(E)"=195476.7023113859, "X(N)"=532749.824259405}, {"Y(E)"=195476.7448714467, "X(N)"=532749.9424745217}, {"Y(E)"=195476.79477031354, "X(N)"=532750.0577839994}, {"Y(E)"=195476.85181105838, "X(N)"=532750.1697327645}, {"Y(E)"=195476.91576856747, "X(N)"=532750.2778790062}, {"Y(E)"=195476.98639042972, "X(N)"=532750.3817959209}, {"Y(E)"=195477.0633979329, "X(N)"=532750.4810733958}, {"Y(E)"=195477.14648716364, "X(N)"=532750.5753196281}, {"Y(E)"=195477.2353302066, "X(N)"=532750.6641626711}, {"Y(E)"=195477.32957643896, "X(N)"=532750.7472519018}, {"Y(E)"=195477.42885391388, "X(N)"=532750.824259405}, {"Y(E)"=195477.53277082852, "X(N)"=532750.8948812673}, {"Y(E)"=195477.64091707027, "X(N)"=532750.9588387763}, {"Y(E)"=195477.75286583535, "X(N)"=532751.0158795213}, {"Y(E)"=195477.8681753131, "X(N)"=532751.0657783881}, {"Y(E)"=195477.98639042972, "X(N)"=532751.1083384489}, {"Y(E)"=195478.10704464413, "X(N)"=532751.1433917385}, {"Y(E)"=195478.22966178932, "X(N)"=532751.1707999178}, {"Y(E)"=195478.35375795135, "X(N)"=532751.1904548189}, {"Y(E)"=195478.47884337942, "X(N)"=532751.2022788732}, {"Y(E)"=195478.60442441847, "X(N)"=532751.2062254163}]}, {"TM array"=[{"Y(E)"=195478.60442441847, "X(N)"=532752.2062254163}, {"Y(E)"=195478.79279597706, "X(N)"=532752.2003056016}, {"Y(E)"=195478.98042411916, "X(N)"=532752.1825695202}, {"Y(E)"=195479.16656836224, "X(N)"=532752.1530871685}, {"Y(E)"=195479.35049407996, "X(N)"=532752.1119748997}, {"Y(E)"=195479.5314754016, "X(N)"=532752.0593949652}, {"Y(E)"=195479.70879807652, "X(N)"=532751.995554874}, {"Y(E)"=195479.88176229317, "X(N)"=532751.9207065736}, {"Y(E)"=195480.04968544078, "X(N)"=532751.8351454564}, {"Y(E)"=195480.2119048034, "X(N)"=532751.7392091928}, {"Y(E)"=195480.36778017535, "X(N)"=532751.6332763993}, {"Y(E)"=195480.51669638773, "X(N)"=532751.5177651446}, {"Y(E)"=195480.65806573626, "X(N)"=532751.3931312986}, {"Y(E)"=195480.79133030074, "X(N)"=532751.259866734}, {"Y(E)"=195480.9159641468, "X(N)"=532751.1184973855}, {"Y(E)"=195481.0314754016, "X(N)"=532750.9695811732}, {"Y(E)"=195481.13740819498, "X(N)"=532750.8137058013}, {"Y(E)"=195481.2333444586, "X(N)"=532750.6514864386}, {"Y(E)"=195481.31890557587, "X(N)"=532750.483563291}, {"Y(E)"=195481.39375387615, "X(N)"=532750.3105990743}, {"Y(E)"=195481.45759396735, "X(N)"=532750.1332763993}, {"Y(E)"=195481.51017390186, "X(N)"=532749.9522950777}, {"Y(E)"=195481.55128617067, "X(N)"=532749.76836936}, {"Y(E)"=195481.58076852243, "X(N)"=532749.582225117}, {"Y(E)"=195481.59850460375, "X(N)"=532749.3945969748}, {"Y(E)"=195481.60442441847, "X(N)"=532749.2062254163}, {"Y(E)"=195481.59850460375, "X(N)"=532749.0178538577}, {"Y(E)"=195481.58076852243, "X(N)"=532748.8302257155}, {"Y(E)"=195481.55128617067, "X(N)"=532748.6440814725}, {"Y(E)"=195481.51017390186, "X(N)"=532748.4601557548}, {"Y(E)"=195481.45759396735, "X(N)"=532748.2791744332}, {"Y(E)"=195481.39375387615, "X(N)"=532748.1018517582}, {"Y(E)"=195481.31890557587, "X(N)"=532747.9288875415}, {"Y(E)"=195481.2333444586, "X(N)"=532747.760964394}, {"Y(E)"=195481.13740819498, "X(N)"=532747.5987450313}, {"Y(E)"=195481.0314754016, "X(N)"=532747.4428696594}, {"Y(E)"=195480.9159641468, "X(N)"=532747.293953447}, {"Y(E)"=195480.79133030074, "X(N)"=532747.1525840985}, {"Y(E)"=195480.65806573626, "X(N)"=532747.019319534}, {"Y(E)"=195480.51669638773, "X(N)"=532746.894685688}, {"Y(E)"=195480.36778017535, "X(N)"=532746.7791744332}, {"Y(E)"=195480.2119048034, "X(N)"=532746.6732416397}, {"Y(E)"=195480.04968544078, "X(N)"=532746.5773053762}, {"Y(E)"=195479.88176229317, "X(N)"=532746.4917442589}, {"Y(E)"=195479.70879807652, "X(N)"=532746.4168959586}, {"Y(E)"=195479.5314754016, "X(N)"=532746.3530558674}, {"Y(E)"=195479.35049407996, "X(N)"=532746.3004759329}, {"Y(E)"=195479.16656836224, "X(N)"=532746.2593636641}, {"Y(E)"=195478.98042411916, "X(N)"=532746.2298813123}, {"Y(E)"=195478.79279597706, "X(N)"=532746.212145231}, {"Y(E)"=195478.60442441847, "X(N)"=532746.2062254163}, {"Y(E)"=195478.4160528599, "X(N)"=532746.212145231}, {"Y(E)"=195478.2284247178, "X(N)"=532746.2298813123}, {"Y(E)"=195478.0422804747, "X(N)"=532746.2593636641}, {"Y(E)"=195477.858354757, "X(N)"=532746.3004759329}, {"Y(E)"=195477.67737343535, "X(N)"=532746.3530558674}, {"Y(E)"=195477.50005076043, "X(N)"=532746.4168959586}, {"Y(E)"=195477.32708654378, "X(N)"=532746.4917442589}, {"Y(E)"=195477.15916339617, "X(N)"=532746.5773053762}, {"Y(E)"=195476.99694403354, "X(N)"=532746.6732416397}, {"Y(E)"=195476.8410686616, "X(N)"=532746.7791744332}, {"Y(E)"=195476.69215244922, "X(N)"=532746.894685688}, {"Y(E)"=195476.55078310068, "X(N)"=532747.019319534}, {"Y(E)"=195476.4175185362, "X(N)"=532747.1525840985}, {"Y(E)"=195476.29288469013, "X(N)"=532747.293953447}, {"Y(E)"=195476.17737343535, "X(N)"=532747.4428696594}, {"Y(E)"=195476.07144064197, "X(N)"=532747.5987450313}, {"Y(E)"=195475.97550437835, "X(N)"=532747.760964394}, {"Y(E)"=195475.88994326108, "X(N)"=532747.9288875415}, {"Y(E)"=195475.8150949608, "X(N)"=532748.1018517582}, {"Y(E)"=195475.7512548696, "X(N)"=532748.2791744332}, {"Y(E)"=195475.6986749351, "X(N)"=532748.4601557548}, {"Y(E)"=195475.65756266628, "X(N)"=532748.6440814725}, {"Y(E)"=195475.62808031452, "X(N)"=532748.8302257155}, {"Y(E)"=195475.6103442332, "X(N)"=532749.0178538577}, {"Y(E)"=195475.60442441847, "X(N)"=532749.2062254163}, {"Y(E)"=195475.6103442332, "X(N)"=532749.3945969748}, {"Y(E)"=195475.62808031452, "X(N)"=532749.582225117}, {"Y(E)"=195475.65756266628, "X(N)"=532749.76836936}, {"Y(E)"=195475.6986749351, "X(N)"=532749.9522950777}, {"Y(E)"=195475.7512548696, "X(N)"=532750.1332763993}, {"Y(E)"=195475.8150949608, "X(N)"=532750.3105990743}, {"Y(E)"=195475.88994326108, "X(N)"=532750.483563291}, {"Y(E)"=195475.97550437835, "X(N)"=532750.6514864386}, {"Y(E)"=195476.07144064197, "X(N)"=532750.8137058013}, {"Y(E)"=195476.17737343535, "X(N)"=532750.9695811732}, {"Y(E)"=195476.29288469013, "X(N)"=532751.1184973855}, {"Y(E)"=195476.4175185362, "X(N)"=532751.259866734}, {"Y(E)"=195476.55078310068, "X(N)"=532751.3931312986}, {"Y(E)"=195476.69215244922, "X(N)"=532751.5177651446}, {"Y(E)"=195476.8410686616, "X(N)"=532751.6332763993}, {"Y(E)"=195476.99694403354, "X(N)"=532751.7392091928}, {"Y(E)"=195477.15916339617, "X(N)"=532751.8351454564}, {"Y(E)"=195477.32708654378, "X(N)"=532751.9207065736}, {"Y(E)"=195477.50005076043, "X(N)"=532751.995554874}, {"Y(E)"=195477.67737343535, "X(N)"=532752.0593949652}, {"Y(E)"=195477.858354757, "X(N)"=532752.1119748997}, {"Y(E)"=195478.0422804747, "X(N)"=532752.1530871685}, {"Y(E)"=195478.2284247178, "X(N)"=532752.1825695202}, {"Y(E)"=195478.4160528599, "X(N)"=532752.2003056016}, {"Y(E)"=195478.60442441847, "X(N)"=532752.2062254163}]}]
  in  "stop":bool
  in  "gmap center":bool
  out "GNSS data info":T3 {"HDOP" scale=0.0..10.0; "PDOP" scale=0.0..10.0; "2D Acc.m" scale=0.0..10.0; "Latitude" format="%.9f"; "Longitude" format="%.9f"; "3D Acc.m" scale=0.0..10.0}
  in  "Gmap Lon":dbl format="%.7f"
  in  "Gmap Lat":dbl format="%.7f"
  in  "gnss tm config":T4(tab)
  out "gnss mode cnt":u32[](array[numeric])
  out "Histogram Graph":cluster{i32[], dbl[]}(graph)
  in  "gnss mode check":bool
  out "Min circle R":dbl format="%.2g"
  out "Points size":i32
  out "loop count":i32
  in  "tm data reset":bool
  in  "arr limit":u32=200
  in  "Ref r size":dbl=1.0 format="%.2f"
  in  "Auto\ncenter":bool
  in  "PinDropMrkr":T5(ring)=enum."red_dot" caption="Pin Drop Marker"
  out "xcenter_TM":dbl
  out "ycenter_TM":dbl
  in  "Lat Dbclk":dbl format="%.11f"
  in  "Lon Dbclk":dbl format="%.11f"
  in  "Center \nupdate s":i32=10000
  in  "zoom":dbl(slide) scale=3.0..20.0
  out "NMEA cluster":T6
  out "Sel NMEA":string
  in  "Sel NMEA type":T7(ring)=enum."$GPGGA"
  in  "GNSS Serial cfg":T8={"Port"="COM10", "rate"=115200}
  in  "GNSS Serial delay":u32=20
  out "Raw NMEA":string
  out "Serial bufferN":u32(graph)
  in  "Data w sel":bool
  in  "baud rate":u32=9600
  in  "NMEA out port":refnum<visa-resource-name> caption="Serial Send Port"
  in  "Write delay ms":u32=900
  out "log path":string
  out "TM array":cluster{"Y(E)":dbl, "X(N)":dbl}[](array[cluster])
  out "error out":errorcluster
  in  "Ntrip accounts":u8(slide) scale=10.0..1.0
  in  "Ntrip accounts":T9(array[cluster])
  in  "update mount point":bool
  in  "Mount points":u16(ring) items=["SONP-RTCM32", "GANS-RTCM32", "GUMC-RTCM32", "DBON-RTCM32", "YONS-RTCM23", "SONP-RTCM23", "GUMC-RTCM23", "GANS-RTCM31", "YONS-CMRx", "SONP-RTCM31", "GUMC-RTCM31", "GANS-RTCM23", "DBON-RTCM23", "DBON-RTCM31", "YONS-RTCM31", "YONS-RTCM32-M5", "VRS-RTCM32-M5", "VRS-RTCM31", "VRS-CMRx", "VRS-CMRplus"]
  out "RTCM recv":string
  out "Current Ntrip client info":T10={"id"="seoul", "pwd"="seoul", "ref pt"="YONS-RTCM32-M5", "address"="gnss.eseoul.go.kr", "port "=2101}
  in  "Ntrip connect":bool
  out "SourceTable recv-str":string
  out "error out 2":errorcluster caption="error out"
  # "GNSS/GPS Test Program"
  # "ver:"
  # "Made by ybbaek https://github.com/yunbum"
  # "RLmodel GNSS-Ntrip client"
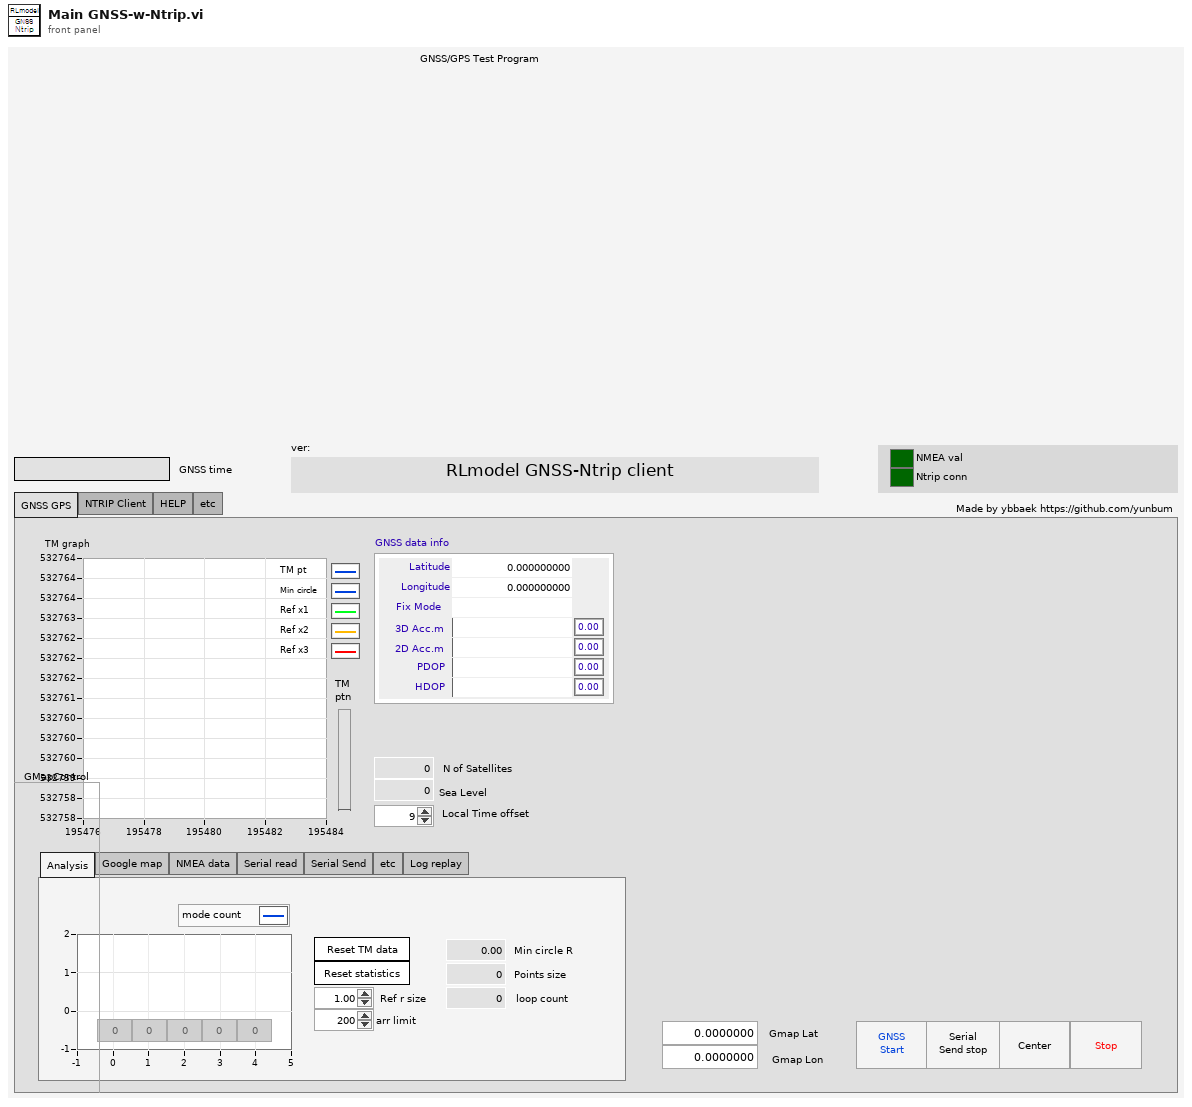
[diagram p1: front panel]
types:
  T1 = enum32{"GNSS GPS", "NTRIP Client", "HELP", "etc"}
  T2 = cluster{"TM array":cluster{"Y(E)":dbl, "X(N)":dbl}[]}[]
  T3 = typedef "ublox-ui_main.ctl" = cluster{"Latitude":dbl, "Longitude":dbl, "Fix Mode":string, "3D Acc.m":dbl, "2D Acc.m":dbl, "PDOP":dbl, "HDOP":dbl}
  T4 = enum32{"Analysis", "Google map", "NMEA data", "Serial read", "Serial Send", "etc", "Log replay"}
  T5 = enum16{"none", "arrow", "blue", "blue_small", "blue_dot", "blue_pushpin", "brown_small", "gray_small", "green", "green_small", "green_dot", "green_pushpin", "green_big_go", "yellow", "yellow_small", "yellow_dot", "yellow_big_pause", "yellow_pushpin", "lightblue", "lightblue_dot", "lightblue_pushpin", "orange", "orange_small", "orange_dot", "pink", "pink_dot", "pink_pushpin", "purple", "purple_small", "purple_dot", "purple_pushpin", "red", "red_small", "red_dot", "red_pushpin", "red_big_stop", "black_small", "white_small"}
  T6 = cluster{"GxGGA":string, "GxGSV":string, "GNRMC":string, "GxTXT":string, "GxGSA":string, "GxGLL":string}
  T7 = enum16{"$GPGSV", "$GLGSV", "$GPGGA", "$GAGSV", "$GBGSV", "$GNGLL", "$GNGGA", "$GNGSA", "$GNRMC", "$GNVTG"}
  T8 = typedef "gnss_config-2.ctl" = cluster{"Port":refnum<visa-resource-name>, "rate":u32}
  T9 = cluster{"id":string, "pwd":string, "ref pt":string, "address":string, "port ":u16}[]
  T10 = cluster{"id":string, "pwd":string, "ref pt":string, "address":string, "port ":u16}
  T11 = typedef "cmd_ini-RW.ctl" = enum16{"ini", "read", "write"}
  T12 = typedef "GNSS-Ntrip config.ctl" = cluster{"Current NtripClient Account":cluster{"id":string, "pwd":string, "ref pt":string, "address":string, "port ":u16}, "Mount points":u16, "Ref r size":dbl, "TMarr limit":i32, "Sel NMEA type":enum16{"$GPGSV", "$GLGSV", "$GPGGA", "$GAGSV", "$GBGSV", "$GNGLL", "$GNGGA", "$GNGSA", "$GNRMC", "$GNVTG"}, "Local Time offset":u32, "Write delay ms":u32, "GNSS Serial delay":u32, "Extra Serial delay":u32, "GNSS Serial cfg":T8, "Ntrip accounts":cluster{"id":string, "pwd":string, "ref pt":string, "address":string, "port ":u16}[]}
  T13 = typedef "cmd_common.ctl" = enum16{"read", "write"}
  T14 = typedef "cmd_ini-add-read.ctl" = enum16{"ini", "add", "read"}
  T15 = typedef "GNSS-Ntrip process val.ctl" = cluster{"GNSS time":string, "Ntrip conn":bool, "NMEA val":bool, "ycenter_TM":dbl, "xcenter_TM":dbl, "TM ref circles":cluster{"Y(E)":dbl, "X(N)":dbl}[], "RTCM recv-str":string, "GNSS Serail buff N":u32, "Sel NMEA type":enum16{"$GPGSV", "$GLGSV", "$GPGGA", "$GAGSV", "$GBGSV", "$GNGLL", "$GNGGA", "$GNGSA", "$GNRMC", "$GNVTG"}, "RTCM recv_sourcetable":string, "NMEA cluster":cluster{"GxGGA":string, "GxGSV":string, "GNRMC":string, "GxTXT":string, "GxGSA":string, "GxGLL":string}, "Sel NMEA str":string, "NMEA recv-str":string}
  T16 = cluster{"Gmap Lat":refnum<vi>, "Gmap Lon":refnum<vi>, "Lat Dbclk":refnum<vi>, "Lon Dbclk":refnum<vi>, "zoom":refnum<vi>, "PinDropMrkr":refnum<vi>}
  T17 = typedef "cmd_RW.ctl" = enum16{"read", "write"}
  T18 = cluster{"Ntrip tcp":bool, "GNSS serial":bool, "RTCM serial":bool, "Extra serial":bool}
  T19 = typedef "gmap_fgv-cmd.ctl" = enum16{"marker type change", "save_image", "coll of points", "zoom n center markers", "add overlay reference", "read", "zoom", "set position by keyword", "set map provider", "map provider update", "create", "add marker", "clear marker", "close"}
  T20 = typedef "NMEA.lvlib/NMEA_LatitudeDirection.ctl" = enum16{"", "North", "South"}
  T21 = typedef "NMEA.lvlib/NMEA_LongitudeDirection.ctl" = enum16{"", "East", "West"}
  T22 = typedef "NMEA.lvlib/NMEA_GPS-Quality.ctl" = enum16{"Invalid", "GPS fix (SPS)", "DGPS fix", "PPS fix", "Real Time Kinematic", "Float RTK", "estimated", "Manual input mode", "Simulation mode"}
  T23 = cluster{"$GPGGA-message_OUT":cluster{"TimeStamp":timestamp, "Latitude":dbl, "Latitude-Direction":T20, "Longitude":dbl, "Longitude-Direction":T21, "GPS-Quality":T22, "N of Satellites":i32, "HDOP":dbl, "Altitude above Mean-Sea-Level":dbl, "Geoidal separation":dbl, "Time since last DGPS update":dbl, "DGPS reference station ID":i32}}
  T24 = cluster{"NA":u32, "valid":u32, "DGPS":u32, "RTK float":u32, "RTK fixed":u32}
  T25 = cluster{"TM array":cluster{"Y(E)":dbl, "X(N)":dbl}[]}
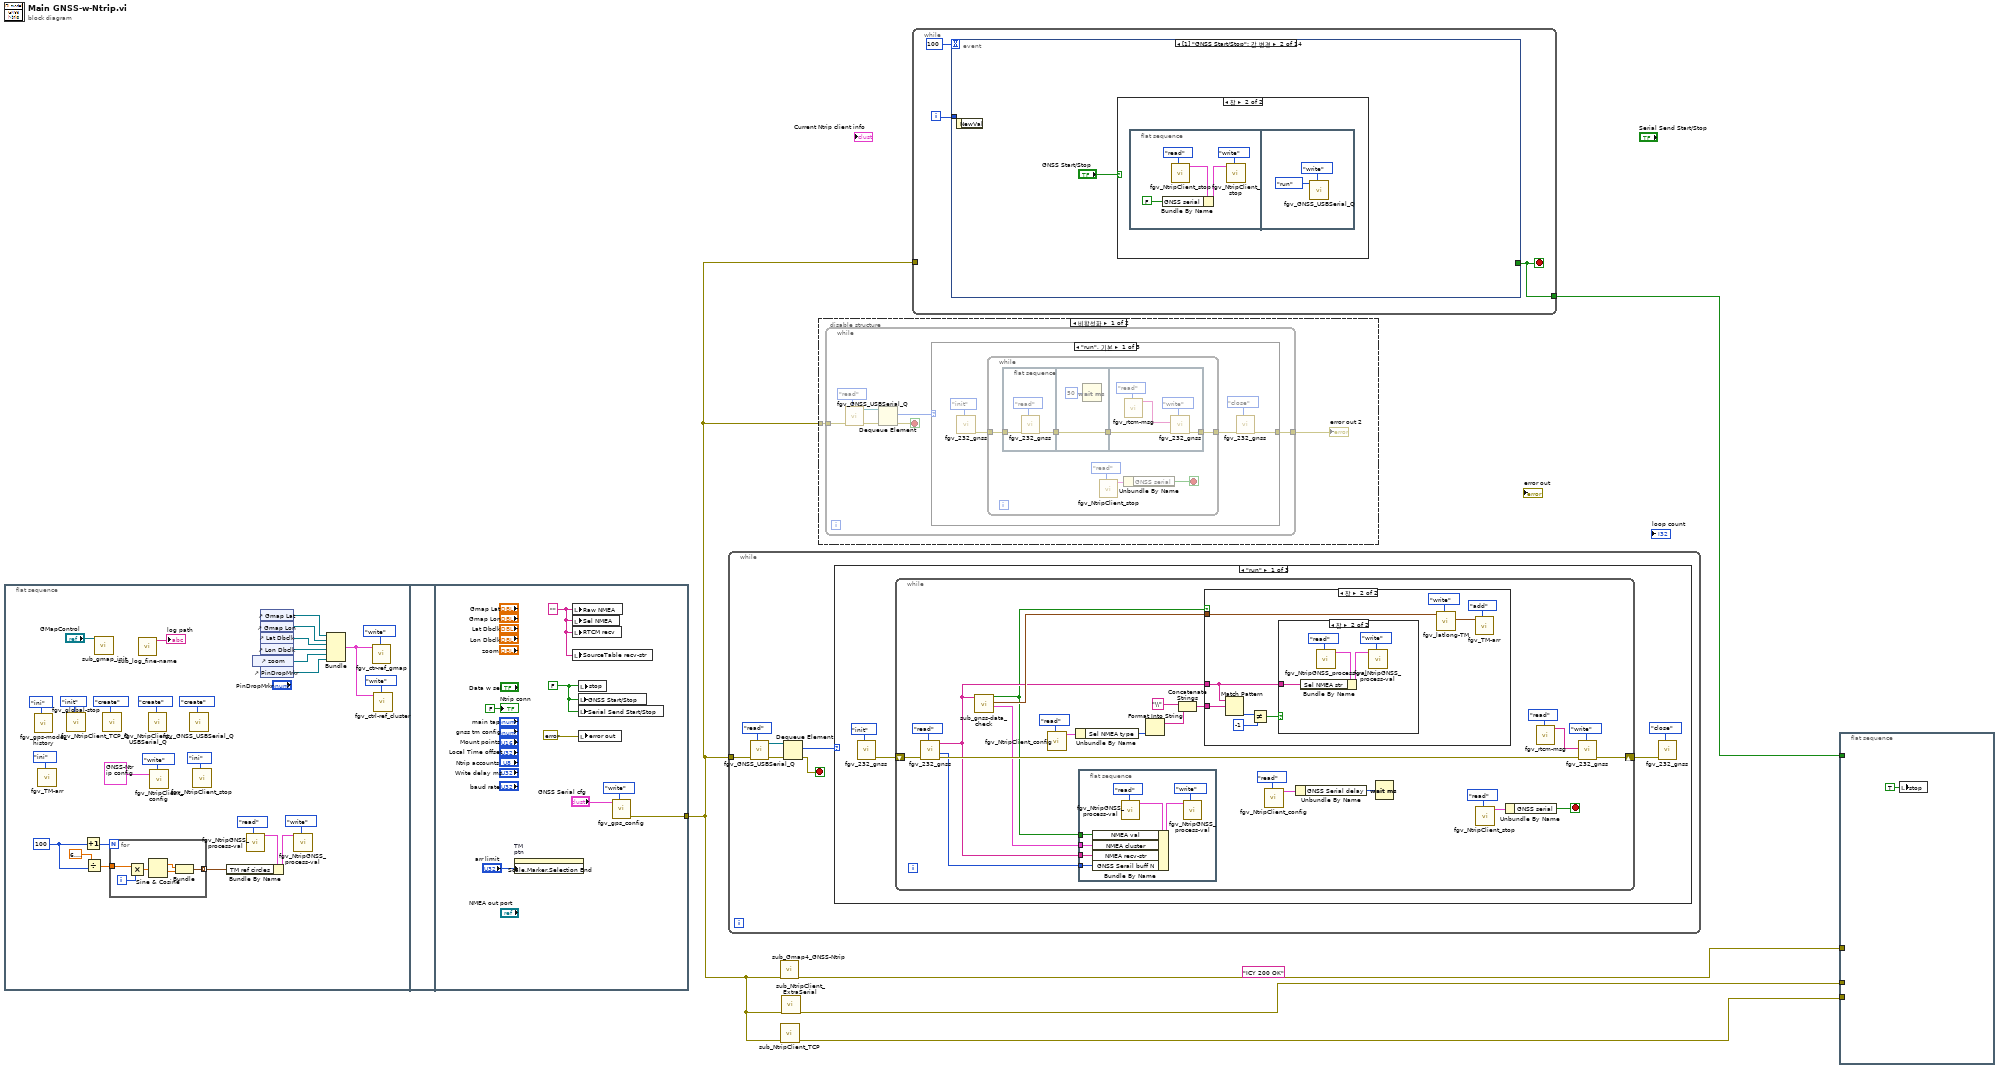
[diagram p0: block diagram]
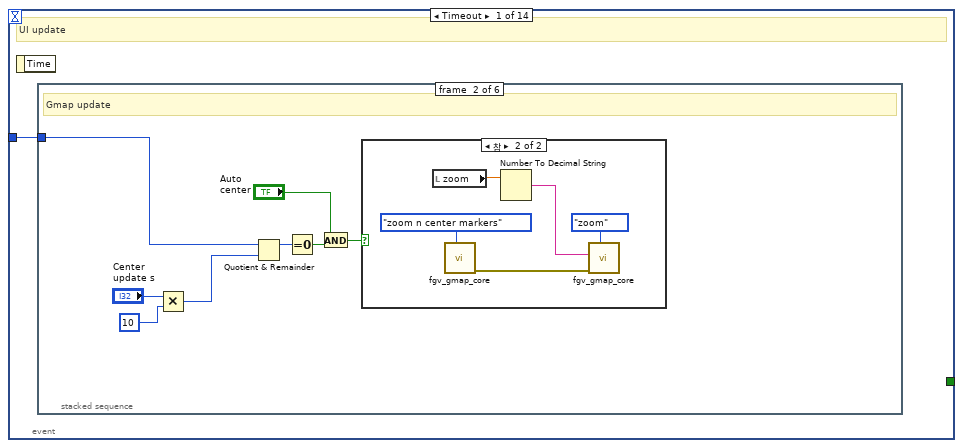
[diagram p9: hidden frame]
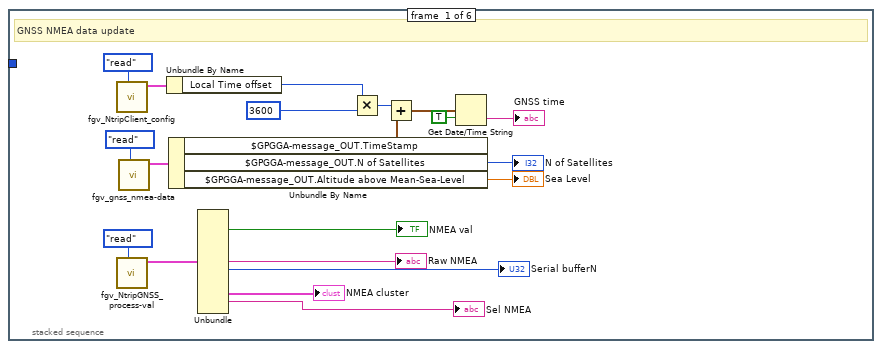
[diagram p10: hidden frame]
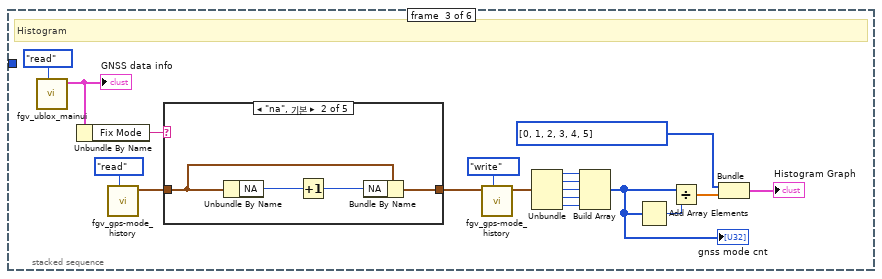
[diagram p12: hidden frame]
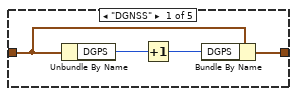
[diagram p13: hidden frame]
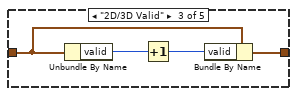
[diagram p14: hidden frame]
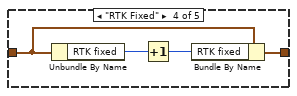
[diagram p15: hidden frame]
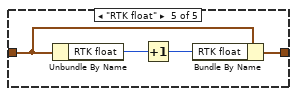
[diagram p16: hidden frame]
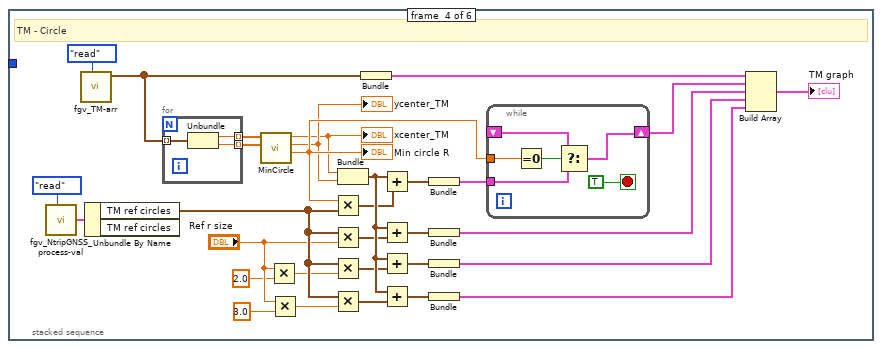
[diagram p17: hidden frame]
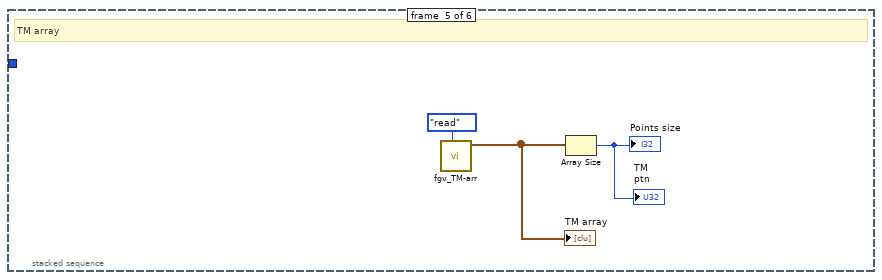
[diagram p18: hidden frame]
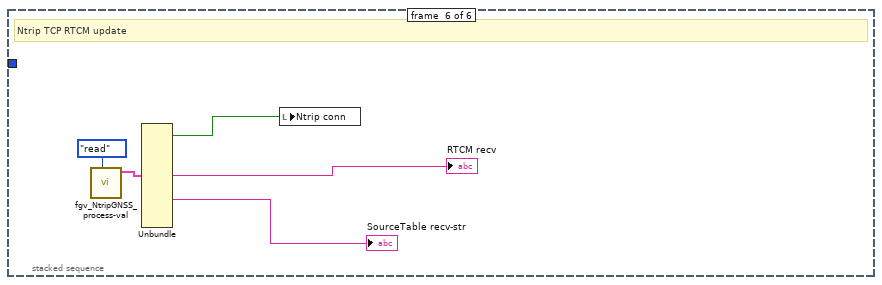
[diagram p19: hidden frame]
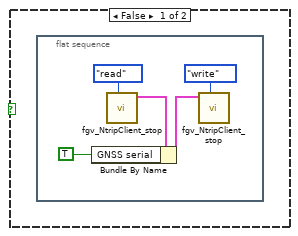
[diagram p20: hidden frame]
diagram:
  (unwired) "ICY 200 OK" ("정규식")
  n1 = flat-sequence {
    tunnel: [w47] -> w1
    frame #0 {
      w15 = 100
      n2 = call "fgv_gps-mode_history.vi"("cmd"=cmd_ini-RW."ini") -> ()  [unwired: 10 in, 1 out]
      n3 = call "fgv_TM-arr.vi"("cmd"=cmd_ini-add-read."ini") -> ()  [unwired: 10 in, 1 out]
      n4 = call "fgv_global-stop.vi"("cmd"=enum16{"init", "stop", "read"}."init") -> ()  [unwired: 10 in, 1 out]
      n5 = Increment(x=w15) -> (x+1=w17:i32)
      n6 = Divide(x=6.283185307179586, y=w15) -> (x/y=w14:dbl)
      n7 = call "sub_gmap_init.vi"("GMapControl"="GMapControl") -> ()  [unwired: 10 in, 1 out]
      n8 = call "fgv_NtripClient_TCP_Q.vi"("cmd"=enum16{"create", "write", "read", "close"}."create") -> ()  [unwired: 9 in, 2 out]
      n9 = for {
        N: w17 -> [_]
        tunnel: w14 -> [w39]
        tunnel: [w35] -> w9 mode=indexing
        i -> [w40]
        n10 = Multiply(x=w39, y=w40) -> (x*y=w38:dbl)
        n11 = Sine & Cosine(0:w38) -> (1:w37:dbl, 2:w36:dbl)
        n12 = Bundle(w37, w36) -> (w35:cluster{dbl, dbl})  [unwired: 1 in]
      }
      n13 = call "sub_log_fine-name.vi"() -> ("log path"=→"log path":string)  [unwired: 11 in]
      n14 = call "fgv_NtripClient_USBSerial_Q.vi"("cmd"=enum16{"create", "write", "read", "close"}."create") -> ()  [unwired: 9 in, 2 out]
      n15 = call "fgv_NtripClient_config.vi"("cmd"=cmd_common."write", "config val"=T12 {"Current NtripClient Account"={"id"="seoul", "pwd"="seoul", "ref pt"="YONS-RTCM32-M5", "address"="gnss.eseoul.go.kr", "port "=2101}, "Mount points"=0, "Ref r size"=1.0, "TMarr limit"=200, "Sel NMEA type"=enum."$GPGGA", "Local Time offset"=9, "Write delay ms"=900, "GNSS Serial delay"=20, "Extra Serial delay"=20, "GNSS Serial cfg"={"Port"="COM10", "rate"=115200}, "Ntrip accounts"=[]}) -> ()  [unwired: 9 in, 1 out]
      n16 = call "fgv_GNSS_USBSerial_Q.vi"("cmd"=enum16{"create", "write", "read", "close"}."create") -> ()  [unwired: 9 in, 2 out]
      n17 = call "fgv_NtripClient_stop.vi"("cmd"=cmd_ini-RW."ini") -> ()  [unwired: 10 in, 1 out]
      n18 = call "fgv_NtripGNSS_process-val.vi"("cmd"=cmd_ini-RW."read") -> ("process val out"=w13:T15)  [unwired: 10 in]
      n19 = Bundle By Name(cluster=w13, "TM ref circles"=w9) -> (w12:T15)
      n20 = control-ref of="zoom"() -> (w28:refnum<vi>)
      n21 = control-ref of="Gmap Lat"() -> (w32:refnum<vi>)
      n22 = control-ref of="Gmap Lon"() -> (w31:refnum<vi>)
      n23 = control-ref of="Lat Dbclk"() -> (w30:refnum<vi>)
      n24 = control-ref of="Lon Dbclk"() -> (w29:refnum<vi>)
      n25 = control-ref of="PinDropMrkr"() -> (w27:refnum<vi>)
      n26 = call "fgv_NtripGNSS_process-val.vi"("cmd"=cmd_ini-RW."write", "process val"=w12) -> ()  [unwired: 9 in, 1 out]
      n27 = Bundle("Gmap Lat"=w32, "Gmap Lon"=w31, "Lat Dbclk"=w30, "Lon Dbclk"=w29, "zoom"=w28, "PinDropMrkr"=w27) -> (w25:T16)  [unwired: 1 in]
      n28 = call "fgv_ctr-ref_gmap.vi"("cmd"=cmd_common."write", "ref in"=w25) -> ()  [unwired: 9 in, 1 out]
      n29 = call "fgv_ctrl-ref_cluster.vi"("cmd"=enum16{"read", "write"}."write", "ref"=w25) -> ()  [unwired: 9 in, 1 out]
    }
    frame #1 {
    }
    frame #2 {
      w42 = "" ("read raw")
      w41 = FALSE ("정지")
      n30 = property on="TM\nptn" class="Slide (엄격한)"("Scale.Marker.Selection End"="arr limit") -> ()  [unwired: 2 in, 2 out]
      n31 = local write "Raw NMEA"(w42) -> ()
      n32 = local write "Sel NMEA"(w42) -> ()
      n33 = local write "RTCM recv"(w42) -> ()
      n34 = local write "SourceTable recv-str"(w42) -> ()
      n35 = local write "GNSS Start/Stop"(w41) -> ()
      n36 = local write "Serial Send Start/Stop"(w41) -> ()
      n37 = local write "stop"(w41) -> ()
      n38 = local write "error out"(errorcluster {"status"=FALSE, "code"=0, "source"=""} ("error out")) -> ()
      n39 = call "fgv_gps_config.vi"("cmd"=enum16{"read", "write"}."write", "GNSS cfg"="GNSS Serial cfg") -> ("error out"=w47:errorcluster)  [unwired: 8 in, 1 out]
      "Ntrip conn" <- FALSE ("ntrip val")
    }
  }
  n40 = while {
    tunnel: w1 -> [w51]
    stop <- w49 stop-if-true
    n41 = call "fgv_GNSS_USBSerial_Q.vi"("cmd"=enum16{"create", "write", "read", "close"}."read", "error in"=w51) -> ("error out"=w50:errorcluster, "queue out"=w54:refnum<queue>)  [unwired: 8 in]
    n42 = Dequeue Element(queue=w54, error in (no error)=w50) -> (element=w52:enum16{"run", "check", "stop"}, error out=w49:errorcluster)  [unwired: 1 in, 2 out]
    n43 = case shown="\"run\"" w52 {
      frame "run" {
        n44 = call "fgv_232_gnss.vi"("cmd"=enum16{"init", "read", "write", "close"}."init") -> ("error out"=w57:errorcluster)  [unwired: 8 in, 2 out]
        n45 = while {
          shift-right: [w72] -> w55
          shift-left: w57 -> [w81]
          stop <- w59 stop-if-true
          n46 = call "fgv_232_gnss.vi"("cmd"=enum16{"init", "read", "write", "close"}."read", "error in"=w81) -> ("error out"=w75:errorcluster, "byte n"=w71:u32, "read_buffer"=w69:string)  [unwired: 7 in]
          n47 = call "sub_gnss-data_check.vi"("gnss str"=w69) -> ("NMEA cluster"=w68:T6, "LatLong"=w80:cluster{dbl, dbl}, "val"=w62:bool)  [unwired: 7 in, 1 out]
          n48 = call "fgv_NtripClient_config.vi"("cmd"=cmd_common."read") -> ("config val out"=w64:T12)  [unwired: 10 in]
          n49 = Unbundle By Name(w64) -> ("Sel NMEA type"=w63:T7)
          n50 = flat-sequence {
            tunnel: w71 -> [w86]
            tunnel: w69 -> [w85]
            tunnel: w68 -> [w84]
            tunnel: w62 -> [w83]
            frame #0 {
              n51 = call "fgv_NtripGNSS_process-val.vi"("cmd"=cmd_ini-RW."read") -> ("process val out"=w90:T15)  [unwired: 10 in]
              n52 = Bundle By Name(cluster=w90, "NMEA val"=w83, "NMEA cluster"=w84, "NMEA recv-str"=w85, "GNSS Serail buff N"=w86) -> (w89:T15)
              n53 = call "fgv_NtripGNSS_process-val.vi"("cmd"=cmd_ini-RW."write", "process val"=w89) -> ()  [unwired: 9 in, 1 out]
            }
          }
          n54 = Format Into String(w63) -> (resulting string=w79:string)  [unwired: 3 in, 1 out]
          n55 = Concatenate Strings("\\" ("string"), w79) -> (w77:string)
          n56 = case shown="참" w62 {
            tunnel: w69 -> [_ w93]
            tunnel: w80 -> [_ w98]
            tunnel: w77 -> [_ w97]
            frame False {
            }
            frame True {
              n57 = Match Pattern(string=w93, regular expression=w97) -> (offset past match=w96:i32)  [unwired: 1 in, 3 out]
              n58 = Not Equal?(x=w96, y=-1) -> (x != y?=w94:bool)
              n59 = case shown="참" w94 {
                tunnel: w93 -> [_ w100]
                frame False {
                }
                frame True {
                  n60 = call "fgv_NtripGNSS_process-val.vi"("cmd"=cmd_ini-RW."read") -> ("process val out"=w104:T15)  [unwired: 10 in]
                  n61 = Bundle By Name(cluster=w104, "Sel NMEA str"=w100) -> (w103:T15)
                  n62 = call "fgv_NtripGNSS_process-val.vi"("cmd"=cmd_ini-RW."write", "process val"=w103) -> ()  [unwired: 9 in, 1 out]
                }
              }
              n63 = call "fgv_latlong-TM.vi"("cmd"=enum16{"write", "read"}."write", "latlong"=w98) -> ("tm out"=w91:cluster{"YE":dbl, "XN":dbl})  [unwired: 8 in, 1 out]
              n64 = call "fgv_TM-arr.vi"("cmd"=cmd_ini-add-read."add", "TM"=w91) -> ()  [unwired: 9 in, 1 out]
            }
          }
          n65 = call "fgv_NtripClient_config.vi"("cmd"=cmd_common."read") -> ("config val out"=w66:T12)  [unwired: 10 in]
          n66 = Unbundle By Name(w66) -> ("GNSS Serial delay"=w70:u32)
          n67 = Wait (ms)(milliseconds to wait=w70) -> ()  [unwired: 1 out]
          n68 = call "fgv_NtripClient_stop.vi"("cmd"=cmd_ini-RW."read") -> ("local stops out"=w61:T18)  [unwired: 10 in]
          n69 = Unbundle By Name(w61) -> ("GNSS serial"=w59:bool)
          n70 = call "fgv_rtcm-msg.vi"("cmd"=cmd_RW."read") -> ("rtcm msg out"=w73:string)  [unwired: 10 in]
          n71 = call "fgv_232_gnss.vi"("cmd"=enum16{"init", "read", "write", "close"}."write", "error in"=w75, "write buff"=w73) -> ("error out"=w72:errorcluster)  [unwired: 6 in, 2 out]
        }
        n72 = call "fgv_232_gnss.vi"("cmd"=enum16{"init", "read", "write", "close"}."close", "error in"=w55) -> ()  [unwired: 7 in, 3 out]
      }
      frame "check" {
      }
      frame "stop", Default {
      }
    }
  }
  n73 = call "sub_Gmap4_GNSS-Ntrip.vi"("error in"=w1) -> ("error out"=w2:errorcluster)  [unwired: 10 in]
  n74 = call "sub_NtripClient_TCP.vi"("error in"=w1) -> ("error out"=w3:errorcluster)  [unwired: 10 in]
  n75 = call "sub_NtripClient_ExtraSerial.vi"("에러 입력(에러 없음)"=w1) -> ("에러 출력"=w4:errorcluster)  [unwired: 10 in]
  n76 = disable-structure shown="비활성화" {
    disable-tunnel: w1 -> [w105 _]
    frame Disabled {
      n77 = while {
        tunnel: w105 -> [w108]
        tunnel: [w107] -> w106
        stop <- w110 stop-if-true
        n78 = call "fgv_GNSS_USBSerial_Q.vi"("cmd"=enum16{"create", "write", "read", "close"}."read", "error in"=w108) -> ("error out"=w112:errorcluster, "queue out"=w111:refnum<queue>)  [unwired: 8 in]
        n79 = Dequeue Element(queue=w111, error in (no error)=w112) -> (element=w109:enum16{"run", "check", "stop"}, error out=w110:errorcluster)  [unwired: 1 in, 2 out]
        n80 = case shown="\"run\", 기본" w109 {
          tunnel: [w114 _ _] -> w107
          frame "run", Default {
            n81 = call "fgv_232_gnss.vi"("cmd"=enum16{"init", "read", "write", "close"}."init") -> ("error out"=w117:errorcluster)  [unwired: 8 in, 2 out]
            n82 = while {
              tunnel: w117 -> [w125]
              tunnel: [w122] -> w115
              stop <- w119 stop-if-true
              n83 = flat-sequence {
                tunnel: w125 -> [w127]
                tunnel: [w126] -> w123
                tunnel: [w129] -> w124
                tunnel: w123 -> [w129]
                tunnel: w124 -> [w134]
                tunnel: [w133] -> w122
                frame #0 {
                  n84 = call "fgv_232_gnss.vi"("cmd"=enum16{"init", "read", "write", "close"}."read", "error in"=w127) -> ("error out"=w126:errorcluster)  [unwired: 7 in, 2 out]
                }
                frame #1 {
                  n85 = Wait (ms)(milliseconds to wait=u32 50 ("대기 시간 (ms)")) -> ()  [unwired: 1 out]
                }
                frame #2 {
                  n86 = call "fgv_rtcm-msg.vi"("cmd"=cmd_RW."read") -> ("rtcm msg out"=w131:string)  [unwired: 10 in]
                  n87 = call "fgv_232_gnss.vi"("cmd"=enum16{"init", "read", "write", "close"}."write", "error in"=w134, "write buff"=w131) -> ("error out"=w133:errorcluster)  [unwired: 6 in, 2 out]
                }
              }
              n88 = call "fgv_NtripClient_stop.vi"("cmd"=cmd_ini-RW."read") -> ("local stops out"=w120:T18)  [unwired: 10 in]
              n89 = Unbundle By Name(w120) -> ("GNSS serial"=w119:bool)
            }
            n90 = call "fgv_232_gnss.vi"("cmd"=enum16{"init", "read", "write", "close"}."close", "error in"=w115) -> ("error out"=w114:errorcluster)  [unwired: 7 in, 2 out]
          }
          frame "check" {
          }
          frame "stop" {
          }
        }
      }
      "error out 2" <- w106
    }
    frame Enabled {
    }
  }
  n91 = while {
    tunnel: w1 -> [_]
    tunnel: [w138] -> w5
    i -> [w136]
    stop <- w138 stop-if-true
    n92 = event shown="[1] \"GNSS Start/Stop\": 값 변경" {
      selector: _ -> [_ _ _ _ _ _ _ _ _ _ _ _ _ _]
      dyn-events: _ -> [_ _ _ _ _ _ _ _ _ _ _ _ _ _]
      timeout: 100 -> [_ _ _ _ _ _ _ _ _ _ _ _ _ _]
      tunnel: [_ _ _ _ _ w281 _ _ _ _ _ _ _ _] -> w138
      tunnel: w136 -> [w139 _ _ _ _ _ _ _ _ _ _ _ _ _]
      event Timeout {
        # "UI update"
        n93 = event-data() -> ()  [unwired: 1 in, 1 out]
        n94 = stacked-sequence {
          tunnel: w139 -> [_ w160 _ _ _ _]
          frame #0 {
            # "GNSS NMEA data update"
            n95 = call "fgv_NtripClient_config.vi"("cmd"=cmd_common."read") -> ("config val out"=w152:T12)  [unwired: 10 in]
            n96 = call "fgv_NtripGNSS_process-val.vi"("cmd"=cmd_ini-RW."read") -> ("process val out"=w145:T15)  [unwired: 10 in]
            n97 = call "fgv_gnss_nmea-data.vi"("cmd"=cmd_common."read") -> ("nmea-data out"=w157:T23)  [unwired: 10 in]
            n98 = Unbundle By Name(w152) -> ("Local Time offset"=w151:u32)
            n99 = Unbundle By Name(w157) -> ("$GPGGA-message_OUT.TimeStamp"=w156:timestamp, "$GPGGA-message_OUT.N of Satellites"=→"N of Satellites":i32, "$GPGGA-message_OUT.Altitude above Mean-Sea-Level"=→"Sea Level":dbl)
            n100 = Unbundle(w145) -> ("NMEA val"=→"NMEA val":bool, "RTCM recv-str"=→"Raw NMEA":string, "GNSS Serail buff N"=→"Serial bufferN":u32, "NMEA cluster"=→"NMEA cluster":T6, "Sel NMEA str"=→"Sel NMEA":string)  [unwired: 8 out]
            n101 = Multiply(x=w151, y=u32 3600) -> (x*y=w159:u32)
            n102 = Add(x=w159, y=w156) -> (x+y=w158:timestamp)
            n103 = Get Date/Time String(seconds (now)=w158, want seconds? (F)=TRUE ("초 보이기? (거짓)")) -> (time string=→"GNSS time":string)  [unwired: 1 in, 1 out]
          }
          frame #1 {
            # "Gmap update"
            n104 = Multiply(x="Center \nupdate s", y=10) -> (x*y=w161:i32)
            n105 = Quotient & Remainder(x=w160, y=w161) -> (x-y*floor(x/y)=w165:i32)  [unwired: 1 out]
            n106 = Equal To 0?(x=w165) -> (x = 0?=w166:bool)
            n107 = And(x="Auto\ncenter", y=w166) -> (x .and. y?=w167:bool)
            n108 = case shown="참" w167 {
              frame False {
              }
              frame True {
                n109 = local read "zoom"() -> (w172:dbl)
                n110 = call "fgv_gmap_core.vi"("cmd"=gmap_fgv-cmd."zoom n center markers") -> ("error out"=w168:errorcluster)  [unwired: 7 in, 3 out]
                n111 = Number To Decimal String(number=w172) -> (decimal integer string=w171:string)  [unwired: 1 in]
                n112 = call "fgv_gmap_core.vi"(7:"cmd"=gmap_fgv-cmd."zoom" ("cmd"), "error in"=w168, 10:"cmd"=w171) -> ()  [unwired: 5 in, 4 out]
              }
            }
          }
          frame #2 {
            # "Histogram"
            n113 = call "fgv_ublox_mainui.vi"("cmd"=cmd_common."read") -> ("MainUI gnss out"=w177:T3)  [unwired: 10 in]
            "GNSS data info" <- w177
            n114 = Unbundle By Name(w177) -> ("Fix Mode"=w178:string)
            n115 = call "fgv_gps-mode_history.vi"("cmd"=cmd_ini-RW."read") -> ("data out"=w179:T24)  [unwired: 10 in]
            n116 = case shown="\"na\", 기본" w178 {
              tunnel: w179 -> [w194 w198 w202 w206 w210]
              tunnel: [w193 w197 w201 w205 w209] -> w180
              frame "DGNSS" {
                n117 = Unbundle By Name(w194) -> ("DGPS"=w192:u32)
                n118 = Increment(x=w192) -> (x+1=w191:u32)
                n119 = Bundle By Name(cluster=w194, "DGPS"=w191) -> (w193:T24)
              }
              frame "na", Default {
                n120 = Unbundle By Name(w198) -> ("NA"=w196:u32)
                n121 = Increment(x=w196) -> (x+1=w195:u32)
                n122 = Bundle By Name(cluster=w198, "NA"=w195) -> (w197:T24)
              }
              frame "2D/3D Valid" {
                n123 = Unbundle By Name(w202) -> ("valid"=w200:u32)
                n124 = Increment(x=w200) -> (x+1=w199:u32)
                n125 = Bundle By Name(cluster=w202, "valid"=w199) -> (w201:T24)
              }
              frame "RTK Fixed" {
                n126 = Unbundle By Name(w206) -> ("RTK fixed"=w204:u32)
                n127 = Increment(x=w204) -> (x+1=w203:u32)
                n128 = Bundle By Name(cluster=w206, "RTK fixed"=w203) -> (w205:T24)
              }
              frame "RTK float" {
                n129 = Unbundle By Name(w210) -> ("RTK float"=w208:u32)
                n130 = Increment(x=w208) -> (x+1=w207:u32)
                n131 = Bundle By Name(cluster=w210, "RTK float"=w207) -> (w209:T24)
              }
            }
            n132 = call "fgv_gps-mode_history.vi"("cmd"=cmd_ini-RW."write", "data"=w180) -> ("data out"=w181:T24)  [unwired: 9 in]
            n133 = Unbundle(w181) -> ("NA"=w182:u32, "valid"=w186:u32, "DGPS"=w185:u32, "RTK float"=w184:u32, "RTK fixed"=w183:u32)
            n134 = Build Array(w182, w186, w185, w184, w183) -> (w190:u32[])
            "gnss mode cnt" <- w190
            n135 = Add Array Elements(numeric array=w190) -> (sum=w188:u32)
            n136 = Divide(x=w190, y=w188) -> (x/y=w189:dbl[])
            n137 = Bundle(i32[] [0, 1, 2, 3, 4, 5], w189) -> (→"Histogram Graph":cluster{i32[], dbl[]})  [unwired: 1 in]
          }
          frame #3 {
            # "TM - Circle"
            n138 = call "fgv_NtripGNSS_process-val.vi"("cmd"=cmd_ini-RW."read") -> ("process val out"=w239:T15)  [unwired: 10 in]
            n139 = call "fgv_TM-arr.vi"("cmd"=cmd_ini-add-read."read") -> ("TM array"=w241:cluster{"Y(E)":dbl, "X(N)":dbl}[])  [unwired: 10 in]
            n140 = Unbundle By Name(w239) -> ("TM ref circles"=w240:cluster{"Y(E)":dbl, "X(N)":dbl}[])  [unwired: 1 out]
            n141 = for {
              tunnel: [w250] -> w216 mode=indexing
              tunnel: [w249] -> w217 mode=indexing
              tunnel: w241 -> [w248] mode=indexing
              n142 = Unbundle(w248) -> ("Y(E)"=w250:dbl, "X(N)"=w249:dbl)
            }
            n143 = call "MinCircle.vi"("y"=w217, "x"=w216) -> ("r"=w226:dbl, "yc"=w219:dbl, "xc"=w218:dbl)  [unwired: 6 in, 1 out]
            "xcenter_TM" <- w218
            "ycenter_TM" <- w219
            "Min circle R" <- w226
            n144 = Multiply(x="Ref r size", y=2.0) -> (x*y=w231:dbl)
            n145 = Multiply(x="Ref r size", y=3.0) -> (x*y=w212:dbl)
            n146 = Multiply(x=w226, y=w240) -> (x*y=w220:cluster{"Y(E)":dbl, "X(N)":dbl}[])
            n147 = Multiply(x=w240, y="Ref r size") -> (x*y=w230:cluster{"Y(E)":dbl, "X(N)":dbl}[])
            n148 = Multiply(x=w240, y=w231) -> (x*y=w229:cluster{"Y(E)":dbl, "X(N)":dbl}[])
            n149 = Multiply(x=w240, y=w212) -> (x*y=w232:cluster{"Y(E)":dbl, "X(N)":dbl}[])
            n150 = Bundle("xc"=w218, "yc"=w219) -> (w233:cluster{"xc":dbl, "yc":dbl})  [unwired: 1 in]
            n151 = Bundle("TM array"=w241) -> (w222:T25)  [unwired: 1 in]
            n152 = Add(x=w233, y=w220) -> (x+y=w221:cluster{dbl, dbl}[])
            n153 = Add(x=w233, y=w230) -> (x+y=w227:cluster{dbl, dbl}[])
            n154 = Add(x=w233, y=w229) -> (x+y=w235:cluster{dbl, dbl}[])
            n155 = Add(x=w233, y=w232) -> (x+y=w234:cluster{dbl, dbl}[])
            n156 = Bundle(w221) -> (w224:cluster{cluster{dbl, dbl}[]})  [unwired: 1 in]
            n157 = Bundle(w227) -> (w228:cluster{cluster{dbl, dbl}[]})  [unwired: 1 in]
            n158 = Bundle(w235) -> (w236:cluster{cluster{dbl, dbl}[]})  [unwired: 1 in]
            n159 = Bundle(w234) -> (w237:cluster{cluster{dbl, dbl}[]})  [unwired: 1 in]
            n160 = while {
              shift-right: [w242] -> w225
              shift-left: _ -> [w244]
              tunnel: w226 -> [w246]
              tunnel: w224 -> [w243]
              stop <- TRUE stop-if-true
              n161 = Equal To 0?(x=w246) -> (x = 0?=w245:bool)
              n162 = Select(t=w244, s=w245, f=w243) -> (s? t:f=w242:cluster{cluster{dbl, dbl}[]})
            }
            n163 = Build Array(w222, w225, w228, w236, w237) -> (→"TM graph":T2)
          }
          frame #4 {
            # "TM array"
            n164 = call "fgv_TM-arr.vi"("cmd"=cmd_ini-add-read."read") -> ("TM array"=w251:cluster{"Y(E)":dbl, "X(N)":dbl}[])  [unwired: 10 in]
            "TM array" <- w251
            n165 = Array Size(array=w251) -> (size(s)=→"Points size" →"TM\nptn":i32)
          }
          frame #5 {
            # "Ntrip TCP RTCM update"
            n166 = call "fgv_NtripGNSS_process-val.vi"("cmd"=cmd_ini-RW."read") -> ("process val out"=w257:T15)  [unwired: 10 in]
            n167 = Unbundle(w257) -> ("Ntrip conn"=w254:bool, "RTCM recv-str"=→"RTCM recv":string, "RTCM recv_sourcetable"=→"SourceTable recv-str":string)  [unwired: 10 out]
            n168 = local write "Ntrip conn"(w254) -> ()
          }
        }
      }
      event "GNSS Start/Stop": Value Change {
        n169 = event-data() -> ()  [unwired: 1 in, 1 out]
        n170 = case shown="참" "GNSS Start/Stop" {
          frame False {
            n171 = flat-sequence {
              frame #0 {
                n172 = call "fgv_NtripClient_stop.vi"("cmd"=cmd_ini-RW."read") -> ("local stops out"=w262:T18)  [unwired: 10 in]
                n173 = Bundle By Name(cluster=w262, "GNSS serial"=TRUE ("Ntrip tcp")) -> (w261:T18)
                n174 = call "fgv_NtripClient_stop.vi"("cmd"=cmd_ini-RW."write", "local stops"=w261) -> ()  [unwired: 9 in, 1 out]
              }
            }
          }
          frame True {
            n175 = flat-sequence {
              frame #0 {
                n176 = call "fgv_NtripClient_stop.vi"("cmd"=cmd_ini-RW."read") -> ("local stops out"=w267:T18)  [unwired: 10 in]
                n177 = Bundle By Name(cluster=w267, "GNSS serial"=FALSE ("Ntrip tcp")) -> (w266:T18)
                n178 = call "fgv_NtripClient_stop.vi"("cmd"=cmd_ini-RW."write", "local stops"=w266) -> ()  [unwired: 9 in, 1 out]
              }
              frame #1 {
                n179 = call "fgv_GNSS_USBSerial_Q.vi"("cmd"=enum16{"create", "write", "read", "close"}."write", "data"=enum16{"run", "check", "stop"}."run") -> ()  [unwired: 8 in, 2 out]
              }
            }
          }
        }
      }
      event "Sel NMEA type": Value Change; "Sel NMEA type": Mouse Down {
        n180 = event-data() -> ()  [unwired: 1 in, 1 out]
      }
      event "GNSS Serial delay": Value Change {
        n181 = event-data() -> ()  [unwired: 1 in, 1 out]
        n182 = call "fgv_NtripClient_config.vi"("cmd"=cmd_common."read") -> ("config val out"=w274:T12)  [unwired: 10 in]
        n183 = Bundle By Name(cluster=w274, "GNSS Serial delay"="GNSS Serial delay") -> (w273:T12)
        n184 = call "fgv_NtripClient_config.vi"("cmd"=cmd_common."write", "config val"=w273) -> ()  [unwired: 9 in, 1 out]
      }
      event "arr limit": Value Change {
        n185 = event-data() -> ()  [unwired: 1 in, 1 out]
        n186 = local read "arr limit"() -> (w277:u32)
        n187 = property on="TM\nptn" class="Slide (엄격한)"("Scale.Marker.Selection End"=w277) -> ()  [unwired: 2 in, 2 out]
      }
      event "stop": Value Change {
        n188 = event-data() -> ()  [unwired: 1 in, 1 out]
        n189 = call "fgv_GNSS_USBSerial_Q.vi"("cmd"=enum16{"create", "write", "read", "close"}."close") -> ()  [unwired: 9 in, 2 out]
        n190 = call "fgv_NtripClient_TCP_Q.vi"("cmd"=enum16{"create", "write", "read", "close"}."close") -> ()  [unwired: 9 in, 2 out]
        n191 = call "fgv_NtripClient_USBSerial_Q.vi"("cmd"=enum16{"create", "write", "read", "close"}."close") -> ()  [unwired: 9 in, 2 out]
        n192 = call "fgv_global-stop.vi"("cmd"=enum16{"init", "stop", "read"}."stop") -> ("val_out"=w281:bool)  [unwired: 10 in]
      }
      event "update mount point": Value Change {
        n193 = event-data() -> ()  [unwired: 1 in, 1 out]
        n194 = call "fgv_NtripClient_TCP_Q.vi"("cmd"=enum16{"create", "write", "read", "close"}."write", "data"=enum16{"run", "check", "stop"}."check") -> ()  [unwired: 8 in, 2 out]
      }
      event "Ntrip accounts": Value Change {
        n195 = event-data() -> ()  [unwired: 1 in, 1 out]
        n196 = Index Array(array="Ntrip accounts", index=0 ("인덱스")) -> ()  [unwired: 1 out]
      }
      event "gmap center": Value Change {
        n197 = event-data() -> ()  [unwired: 1 in, 1 out]
        n198 = call "fgv_gmap_core.vi"("cmd"=gmap_fgv-cmd."zoom n center markers") -> ("error out"=w287:errorcluster)  [unwired: 7 in, 3 out]
        n199 = local read "zoom"() -> (w290:dbl)
        n200 = Number To Decimal String(number=w290) -> (decimal integer string=w289:string)  [unwired: 1 in]
        n201 = call "fgv_gmap_core.vi"(7:"cmd"=gmap_fgv-cmd."zoom" ("cmd"), "error in"=w287, 10:"cmd"=w289) -> ()  [unwired: 5 in, 4 out]
      }
      event "Ntrip connect": Value Change {
        n202 = event-data() -> ()  [unwired: 1 in, 1 out]
        n203 = case shown="참" "Ntrip connect" {
          frame False {
            n204 = call "fgv_NtripClient_stop.vi"("cmd"=cmd_ini-RW."read") -> ("local stops out"=w295:T18)  [unwired: 10 in]
            n205 = Bundle By Name(cluster=w295, "Ntrip tcp"=TRUE) -> (w294:T18)
            n206 = call "fgv_NtripClient_stop.vi"("cmd"=cmd_ini-RW."write", "local stops"=w294) -> ()  [unwired: 9 in, 1 out]
          }
          frame True {
            n207 = flat-sequence {
              frame #0 {
                n208 = call "fgv_NtripClient_stop.vi"("cmd"=cmd_ini-RW."read") -> ("local stops out"=w302:T18)  [unwired: 10 in]
                n209 = Bundle By Name(cluster=w302, "Ntrip tcp"=FALSE) -> (w301:T18)
                n210 = call "fgv_NtripClient_stop.vi"("cmd"=cmd_ini-RW."write", "local stops"=w301) -> ()  [unwired: 9 in, 1 out]
              }
              frame #1 {
                n211 = call "fgv_NtripClient_TCP_Q.vi"("cmd"=enum16{"create", "write", "read", "close"}."write", "data"=enum16{"run", "check", "stop"}."run") -> ()  [unwired: 8 in, 2 out]
              }
            }
          }
        }
      }
      event "tm data reset": Value Change {
        # "TM GPS data array reset"
        n212 = event-data() -> ()  [unwired: 1 in, 1 out]
        n213 = case shown="참" "tm data reset" {
          frame False {
          }
          frame True {
            n214 = call "fgv_TM-arr.vi"("cmd"=cmd_ini-add-read."ini") -> ()  [unwired: 10 in, 1 out]
          }
        }
      }
      event "zoom": Value Change {
        n215 = event-data() -> ()  [unwired: 1 in, 1 out]
        n216 = local read "zoom"() -> (w308:dbl)
        n217 = Number To Decimal String(number=w308) -> (decimal integer string=w307:string)  [unwired: 1 in]
        n218 = call "fgv_gmap_core.vi"(7:"cmd"=gmap_fgv-cmd."zoom" ("cmd"), 10:"cmd"=w307) -> ()  [unwired: 6 in, 4 out]
      }
      event "gnss mode check": Value Change {
        n219 = event-data() -> ()  [unwired: 1 in, 1 out]
        n220 = call "fgv_gps-mode_history.vi"("cmd"=cmd_ini-RW."ini") -> ()  [unwired: 10 in, 1 out]
      }
      event Value Change {
        n221 = event-data() -> ()  [unwired: 1 in, 1 out]
        n222 = local read "GNSS Serial cfg"() -> (w311:T8)
        n223 = call "fgv_gps_config.vi"("cmd"=enum16{"read", "write"}."write", "GNSS cfg"=w311) -> ()  [unwired: 8 in, 2 out]
      }
    }
  }
  n224 = flat-sequence {
    tunnel: w5 -> [_]
    tunnel: w4 -> [_]
    tunnel: w3 -> [_]
    tunnel: w2 -> [_]
    frame #0 {
      n225 = local write "stop"(TRUE ("stop")) -> ()
    }
  }
